vi "Dashboard Main.vi"() -> ()   [LabVIEW 2015]
uses:
  C/Program Files (x86)/National Instruments/LabVIEW 2015/examples/FRC/roboRIO/Vision/2016 Vision Example/Vision Support Code/Camera Types.ctl
  <vilib>/Rock Robotics/WPI/Camera/WPI_CameraSettings Read MJPG.ctl
  <vilib>/Rock Robotics/WPI/Camera/WPI_CameraImageSize.ctl
  <vilib>/Utility/miscctls.llb/LVRowAndColumnTypeDef.ctl
  <vilib>/event_ctls.llb/eventvkey.ctl
  <vilib>/Rock Robotics/WPI/Dashboard/WPI_DashboardLogging Global.vi
  <vilib>/Rock Robotics/Network Tables/NT Write Boolean.vi
  <vilib>/Rock Robotics/Network Tables/NT Read Numeric Array.vi
  <vilib>/Utility/config.llb/Write Key (String).vi
  <vilib>/Utility/config.llb/Write Key (I32).vi
  <vilib>/Utility/config.llb/NI_LVConfig.lvlib
  <vilib>/vision/NI_Vision_Development_Module.lvlib
panel:
  in  "Vision":u16(ring)=1 items=["Camera Off", "USB Camera SW", "USB Camera HW", "IP Camera"]
  out "Camera IP 2":string
  in  "Rec Mode 2":enum32{"Stop", "Record", "Playback"}(radio)
  out "Original Image":T1(plugin-control)
  out "Sorted Particle Scores":T2(array[cluster]) {"Moment Factor" format="%#_3g"; "Aspect Ratio" format="%#_3g"; "Area to CH" format="%#_3g"; "X" format="%#_3g"; "Y" format="%#_3g"}
  out "Detected Targets":T3(array[cluster]) {"Normalized Rect"."Numeric 5" format="%#_2g"; "Normalized Rect"."Numeric 3" format="%#_2g"; "Normalized Rect"."Numeric 2" format="%#_2g"; "Normalized Rect"."Numeric" format="%#_2g"}
  in  "TCP":refnum<k5>
  in  "Rec Mode":enum32{"Stop", "Record", "Playback"}(radio)
  in  "Vision - Dissabled Control":u16(ring)=1 items=["Camera Off", "USB Camera SW", "USB Camera HW", "IP Camera"]
  out "Camera IP":string
  out "Image Message":string="Timeout in Camera Communications"
  in  "Dashboard Tab":T4(tab)
  in  "ACTIVE CAMERA":bool=TRUE
  out "Target Horizontal Degrees":dbl(knob) scale=-30.0..30.0
  out "Target Vertical Angle":dbl(knob) scale=-30.0..30.0
  out "Target Visible":bool
  in  "Camera Address 2":string="USB 0"
  in  "Camera Settings":T5={"fps"=30, "compression"=30, "Image Size"=enum."640x480"}
  out "Auton Mode":string
  in  "Select Auto":string(combo)
  out "NT Connection":bool
  in  "Camera Settings":T7={"Frame Rate"=30, "Compression"=30, "Size"=1} {"Frame Rate" scale=1.0..30.0; "Size" items=["640x480", "320x240", "160x120"]}
  out "MotorChart R":cluster{"Numeric":dbl, "Numeric":dbl}(graph)
  out "MotorChart L":T8(graph)
  out "MotorSliders R":cluster{"MotorSlide1":dbl, "MotorSlide2":dbl} {"MotorSlide2" scale=-1.0..1.0 scale format="%#_2e"; "MotorSlide1" scale=-1.0..1.0 scale format="%#_2e"}
  out "MotorSliders L":T9 {"MotorSlide4 2" scale=0.0..14.0 scale format="%#_2e"; "MotorSlide2" scale=-1.0..1.0 scale format="%#_2e"; "MotorSlide1" scale=-1.0..1.0 scale format="%#_2e"}
  out "Gyro":dbl(knob) scale=0.0..360.0
  out "JS1 Z":dbl(slide) scale=-1.0..1.0 scale format="%#_2e"
  out "JS1 Graph":cluster{"X":dbl, "Y":dbl}[](graph)
  out "JS1 Buttons":T10
  out "JS2 Z":dbl(slide) scale=-1.0..1.0 scale format="%#_2e"
  out "JS2 Graph":cluster{"X":dbl, "Y":dbl}[](graph)
  out "JS2 Buttons":T10
  out "Mode":T11(ring)=enum."Auto Disabled"
  in  "DB Camera Config":bool
  out "fps":dbl format="%#.1g"
  out "Mbps":dbl format="%#.1g"
  out "Mbps LED":bool
  in  "DB/String 9":string
  in  "DB/String 8":string
  in  "DB/String 7":string
  in  "DB/String 6":string
  in  "DB/String 5":string
  in  "DB/String 4":string
  in  "DB/String 3":string
  in  "DB/String 2":string
  in  "DB/String 1":string
  in  "DB/String 0":string
  in  "DB/Slider 0":dbl(slide) scale=0.0..5.0
  in  "DB/Slider 1":dbl(slide) scale=0.0..5.0
  in  "DB/Slider 2":dbl(slide) scale=0.0..5.0
  in  "DB/Slider 3":dbl(slide) scale=0.0..5.0
  out "DB/LED 3":bool
  out "DB/LED 2":bool
  out "DB/LED 1":bool
  out "DB/LED 0":bool
  in  "DB/Button 3":bool
  in  "DB/Button 2":bool
  in  "DB/Button 1":bool
  in  "DB/Button 0":bool caption="New Name"
  in  "LED Color":T12={"Hue"={45.0, 125.0}, "Sat"={0.0, 255.0}, "Val"={250.0, 255.0}} {"Hue" scale=0.0..255.0 scale format="%#_3g"}
  in  "Std Devs for Cal":cluster{"H":dbl, "S":dbl, "V":dbl}={"H"=4.0, "S"=6.0, "V"=4.0}
  in  "Min Score Thresh":i32=60
  out "Highest Avg Score":dbl format="%#_3g"
  in  "Anno Limit":dbl=75.0
  out "Qualified Particles":i32
  out "Masked":T1(plugin-control)
  in  "Green BCG Values (Brightness 1)":T13={"Brightness"=100.0, "Contrast"=45.0, "Gamma"=1.0}
  in  "Annotate":bool=TRUE
  in  "Asp Rat FFact":dbl=1.0
  in  "Emphasize Limit Tests":bool=TRUE
  in  "Camera Type":T14=enum."MS HD3000 640x480"
  in  "Test Slider":dbl(slide) scale=0.0..100.0 scale format="%#_3g"
  in  "On/Off":bool caption="Solenoid"
  in  "Test Name":u16(ring) items=["Select the test to run..."]
  in  "Test Tree":string(tree)
  in  "Motor":cluster{"Value":dbl, "Enable":bool} {"Value" scale=-1.0..1.0 scale format="%#_3g"}
  out "Progress":T15 {"Test Progress" scale=0.0..100.0}
  in  "Rev/Fwd":cluster{"Forward":bool, "Reverse":bool}
  in  "Test Ring":u16(ring) items=["Monochrome", "Color"]
  out "Cmd Status":string
  in  "Execute Command":bool
  in  "Command Params":string[][](table)
  in  "Command Selection":i32(listbox)
  in  "CheckList":i32(listbox)
  out "Tree":string(tree)
  out "Camera Image":T1(plugin-control)
  out "Background":bool
  # "Density Profile"
  # "Left"
  # "Front"
  # "Right"
  # "Battery"
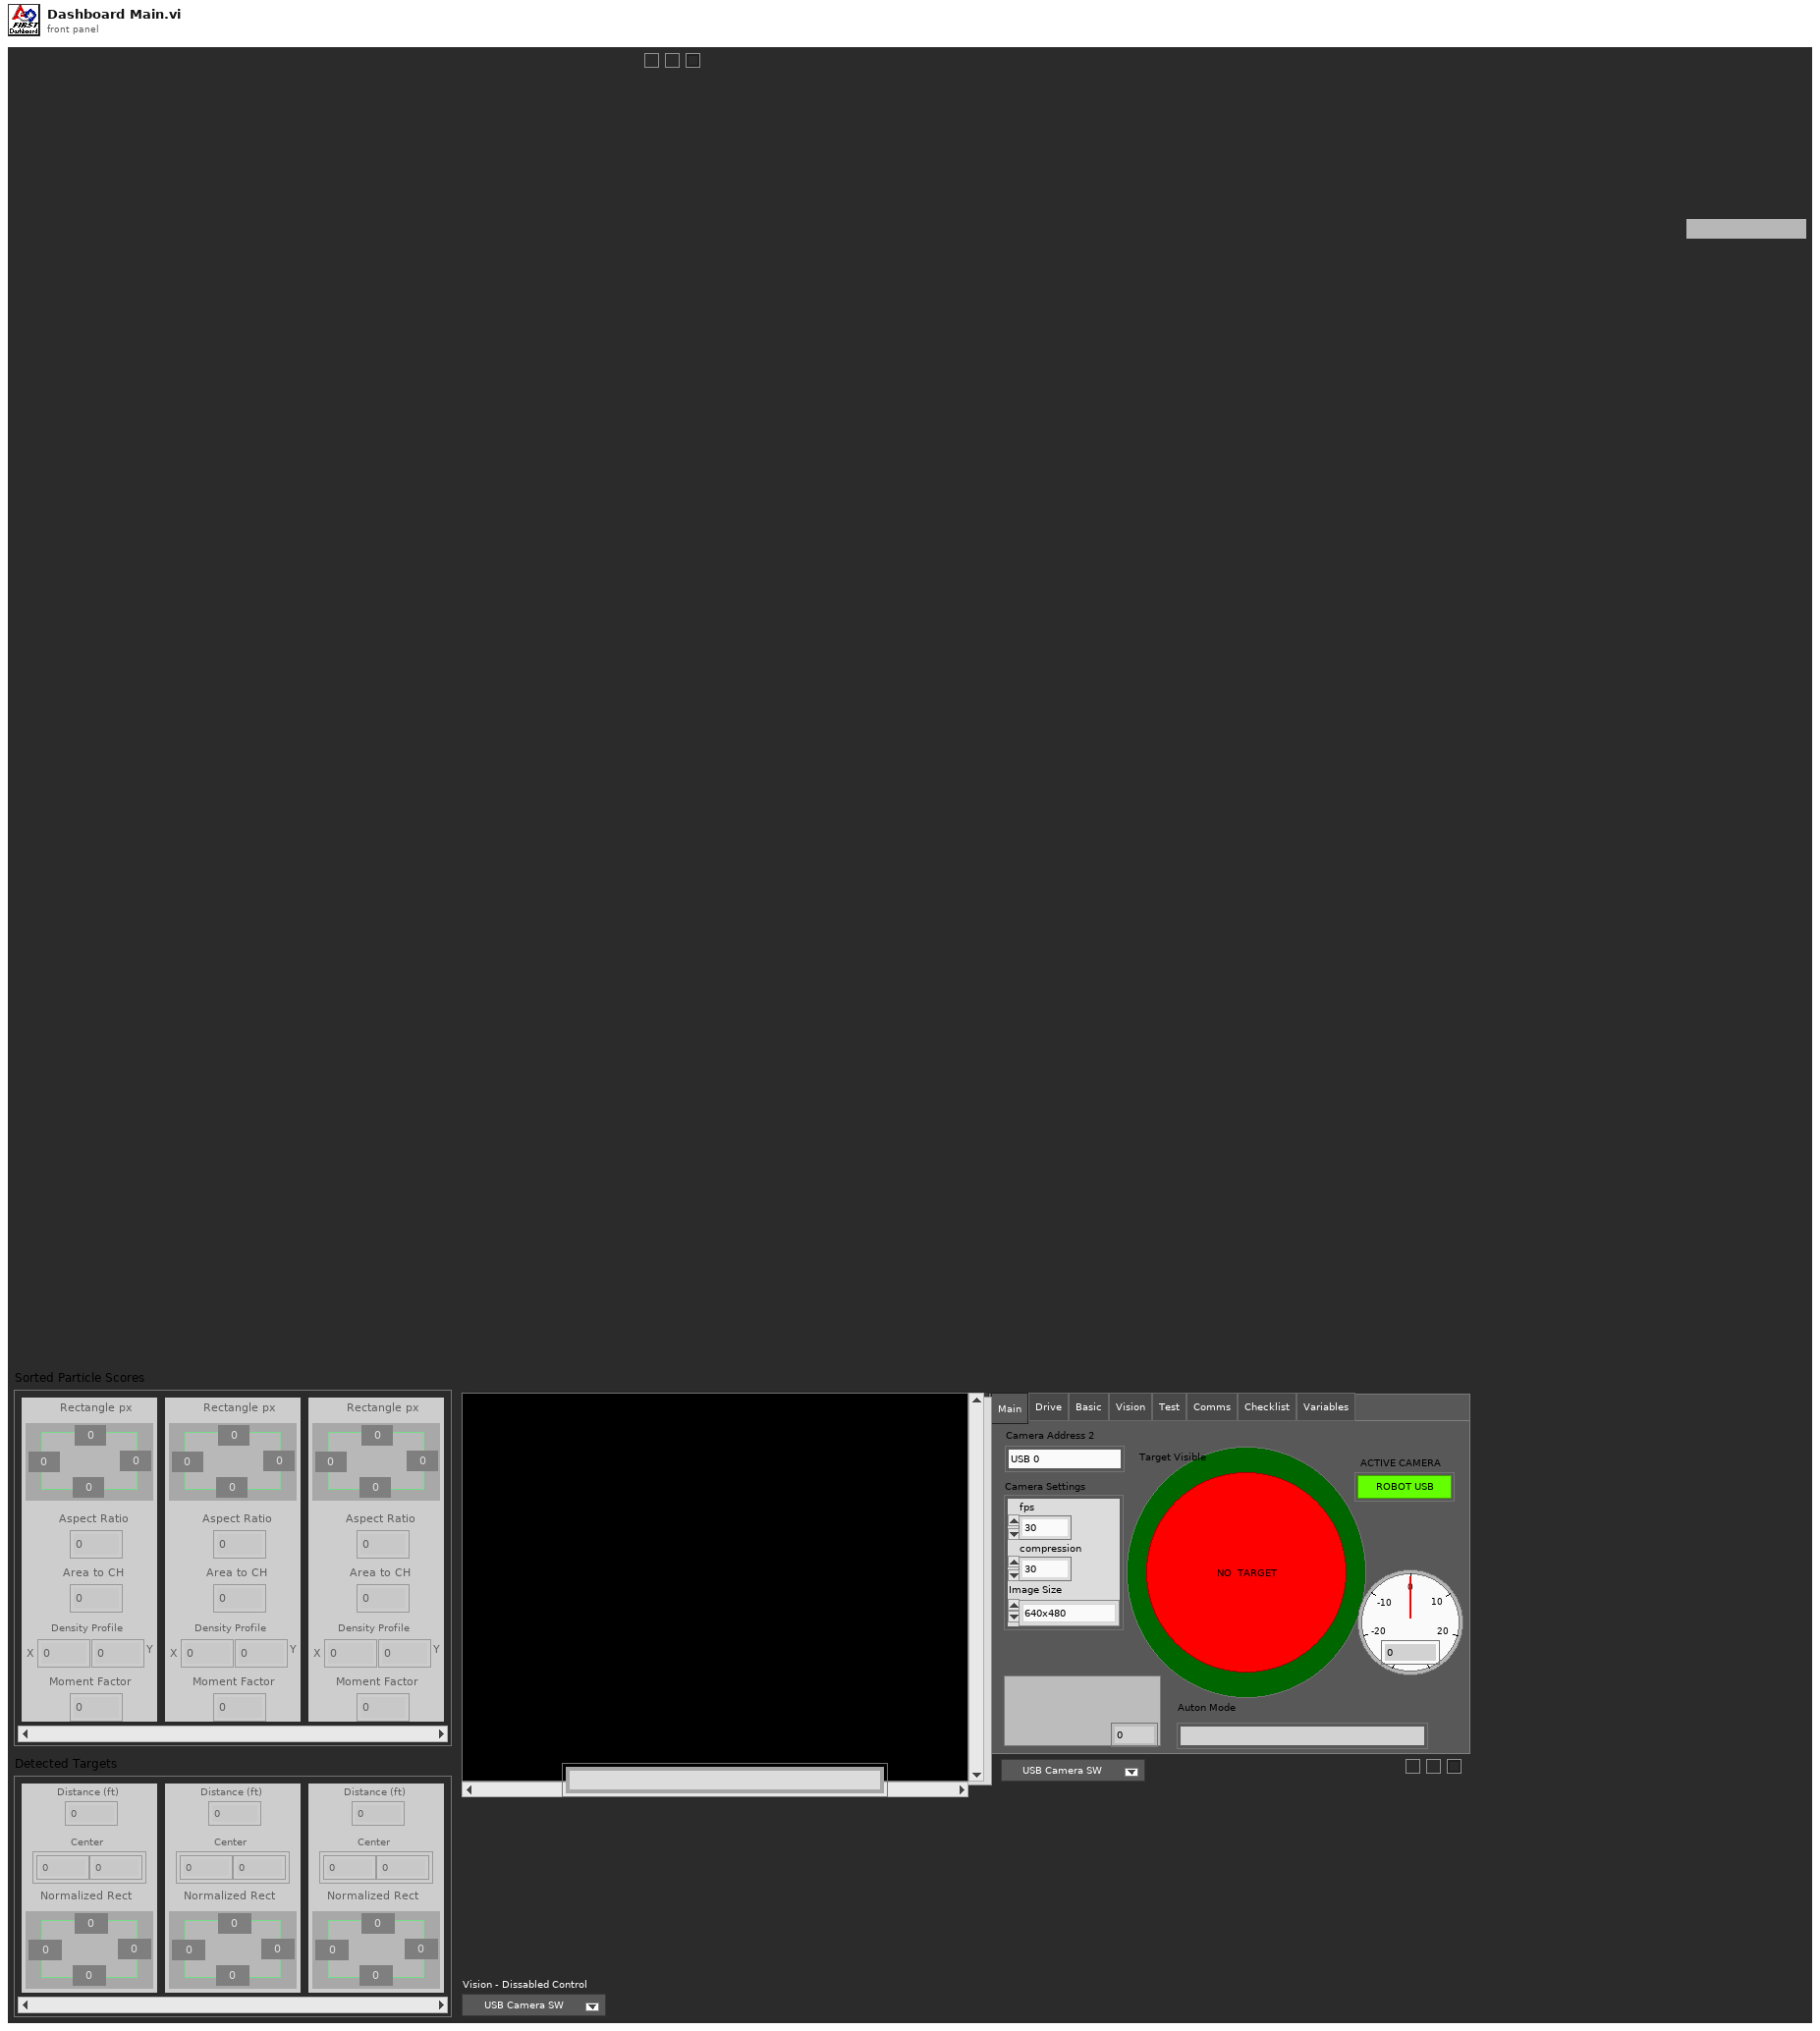
[diagram p1: front panel]
types:
  T1 = typedef "IMAQ Image.ctl" = refnum<image>
  T2 = cluster{"Rectangle px":cluster{"Numeric":dbl, "Numeric 2":dbl, "Numeric 3":dbl, "Numeric 5":dbl}, "Aspect Ratio":dbl, "Area to CH":dbl, "X":dbl, "Y":dbl, "Moment Factor":dbl}[]
  T3 = cluster{"Distance (ft)":dbl, "Center":cluster{dbl, dbl}, "Normalized Rect":cluster{"Numeric":dbl, "Numeric 2":dbl, "Numeric 3":dbl, "Numeric 5":dbl}}[]
  T4 = enum32{"Main", "Drive", "Basic", "Vision", "Test", "Comms", "Checklist", "Variables"}
  T5 = typedef "WPI_CameraSettings Read MJPG.ctl" = cluster{"fps":i32, "compression":i32, "Image Size":T6}
  T6 = typedef "WPI_CameraImageSize.ctl" = enum16{"640x480", "320x240", "160x120", "Custom"}
  T7 = cluster{"Frame Rate":i32, "Compression":i32, "Size":u16}
  T8 = cluster{"Numeric":dbl, "Numeric":dbl, "Battery V":dbl}
  T9 = cluster{"MotorSlide1":dbl, "MotorSlide2":dbl, "MotorSlide4 2":dbl}
  T10 = cluster{bool, bool, bool, bool, bool, bool, bool, bool, bool, bool, bool, bool}
  T11 = enum8{"Tele-Op Disabled", "Tele-Op Enabled", "Auto Disabled", "Auto Enabled", "Test Disabled", "Test Enabled", "Disconnected", "No Code", "E-Stop"}
  T12 = cluster{"Hue":cluster{dbl, dbl}, "Sat":cluster{dbl, dbl}, "Val":cluster{dbl, dbl}}
  T13 = cluster{"Brightness":sgl, "Contrast":sgl, "Gamma":sgl}
  T14 = typedef "Camera Types.ctl" = enum16{"206", "1011", "1013", "MS HD3000 square", "MS HD3000 640x480"}
  T15 = cluster{"Test Progress":u8, "Test Progress Text":string}
  T16 = typedef "Particle Parameters" = i32
  T17 = typedef "Image Type" = u32
  T18 = cluster{"IDs":cluster{"RPC field ID":u16, "Unique ID":u16}, "String":string}
  T19 = enum32{"Drive", "Basic", "Custom", "Test", "Checklist", "Variables"}
  T20 = cluster{"Camera Image":refnum<vi>, "Dashboard Tab":refnum<vi>, "Background":refnum<vi>, "Vision - Dissabled Control":refnum<vi>, "Rec Mode":refnum<vi>, "Test Slider":refnum<vi>, "On/Off ":refnum<vi>, "Test Ring":refnum<vi>, "Rev/Fwd":refnum<vi>, "Test Name":refnum<vi>, "Motor":refnum<vi>, "Progress":refnum<vi>, "CheckList":refnum<vi>, "Tree":refnum<vi>, "Test Tree":refnum<vi>, "Command Params":refnum<vi>, "Command Selection":refnum<vi>, "Execute Command":refnum<vi>, "Cmd Status":refnum<vi>}
  T21 = cluster{cluster{dbl, dbl}, cluster{dbl, dbl}, cluster{dbl, dbl}}
  T22 = cluster{"Bounding box":cluster{"left":dbl, "top":dbl, "right":dbl, "bottom":dbl}, "Aspect Ratio":dbl, "Area to CH":dbl, "X Mask":dbl, "Y Mask":dbl, "Moment":dbl}[]
  T23 = cluster{"Rectangle":cluster{"Numeric":dbl, "Numeric 2":dbl, "Numeric 3":dbl, "Numeric 5":dbl}, "L":dbl, "Area to CH":dbl, "X":dbl, "Y":dbl, "Moment Factor":dbl}[]
  T24 = cluster{"Distance (ft)":dbl, "Center":cluster{dbl, dbl}, "Normalized Rect":cluster{"Numeric":dbl, "Numeric 2":dbl, "Numeric 3":dbl, "Numeric 5":dbl}}
  T25 = cluster{"Rectangle":cluster{"Numeric":dbl, "Numeric 2":dbl, "Numeric 3":dbl, "Numeric 5":dbl}, "L":dbl, "Area to CH":dbl, "X":dbl, "Y":dbl, "Moment Factor":dbl}
  T26 = cluster{"Numeric":dbl, "Numeric 2":dbl, "Numeric 3":dbl, "Numeric 5":dbl}
  T27 = cluster{"Error Strings":string, "Disable Counts":cluster{u16, u16}, "Rail Faults":cluster{u16, u16, u16}, "Robot IP":string, "DB Mode":u8, "Event Info":cluster{"Name":string, "Type":u8, "Number":u16, "Replay":u8}, "Camera Addr":string}
  T28 = cluster{"Storage":cluster{"Disk Free":u64, "RAM Block":u32, "RAM free":u32}, "CPU Utilization":cluster{"CPU % ISR":sgl, "CPU % Time Crit":sgl, "CPU % Timed Str":sgl, "CPU % High":sgl, "CPU % Above":sgl, "CPU % Normal":sgl, "CPU % Low":sgl}, "CAN":cluster{"% Bus Utilization":sgl, "Bus Off Cnt":u32, "TX_FIFO Full Cnt":u32, "Receive Error Cnt":u8, "Transmit Error Cnt":u8}, "HID":cluster{"HID Outputs":u32, "Rumble Low":u16, "Rumble High":u16}[]}
  T29 = cluster{"Status bits":cluster{"Test Mode":bool, "Autonomous":bool, "Enabled":bool, "Code Start":bool, "Brownout":bool, "Reserved 2":bool, "Reserved 3":bool, "E-Stop":bool}, "Code Trace":cluster{"Disabled":bool, "TeleOp":bool, "Auto":bool, "Test":bool}, "Controller Type":enum16{"unknown", "cRIO", "roboRio"}, "Code?":enum16{"unknown", "noCode", "code"}, "Battery V":dbl}
  T30 = cluster{"Control Bits":cluster{"TestMode":bool, "Autonomous":bool, "Enabled":bool, "FMS Present":bool, bool, bool, bool, "E-Stop":bool}, "Team Station ":u8, "Countdown":sgl, "Joystick Values":cluster{"Axes":dbl[], "Buttons":bool[], "POVs":i16[]}[]}
  T31 = cluster{"Axes":dbl[], "Buttons":bool[], "POVs":i16[]}[]
  T32 = cluster{"Axes":dbl[], "Buttons":bool[], "POVs":i16[]}
  T33 = cluster{"Buttons[0]":bool, "Buttons[1]":bool, "Buttons[2]":bool, "Buttons[3]":bool, "Buttons[4]":bool, "Buttons[5]":bool, "Buttons[6]":bool, "Buttons[7]":bool, "Buttons[8]":bool, "Buttons[9]":bool, "Buttons[10]":bool, "Buttons[11]":bool}
  T34 = typedef "NI_LVConfig.lvlib/Config Data RefNum.ctl" = refnum<k1>
  T35 = cluster{"Operation":enum16{"Update", "Clear"}, "Color Box":u32}[]
  T36 = typedef "eventvkey.ctl" = enum16{"ASCII", "Enter", "Return", "Shift", "Ctrl", "Alt", "Cmd", "Opt", "Caps", "NumLock", "Clear", "Break", "Up", "Down", "Left", "Right", "Insert", "Delete", "Home", "End", "PageUp", "PageDown", "Escape", "Help", "Pause", "ScrollLock", "F1", "F2", "F3", "F4", "F5", "F6", "F7", "F8", "F9", "F10", "F11", "F12", "F13", "F14", "F15", "F16", "F17", "F18", "F19", "F20", "F21", "F22", "F23", "F24", "Play", "VolumeUp", "VolumeDown", "Mute", "Two Byte Char"}
  T37 = cluster{"Image Size":bool, "Image Type":bool, "Pixel Value":bool, "ROI Information":bool, "Zoom Factor":bool}
  T38 = enum8{"Enabled", "Disabled", "Disabled and Grayed Out"}
  T39 = cluster{"Operation":enum16{"Update", "Clear"}, "Color Box":u32}
  T40 = typedef "LVRowAndColumnTypeDef.ctl" = cluster{"Row":i32, "Column":i32}
  T41 = cluster{"Shift":bool, "Ctrl":bool, "Alt":bool, "Cmd":bool, "Opt":bool}
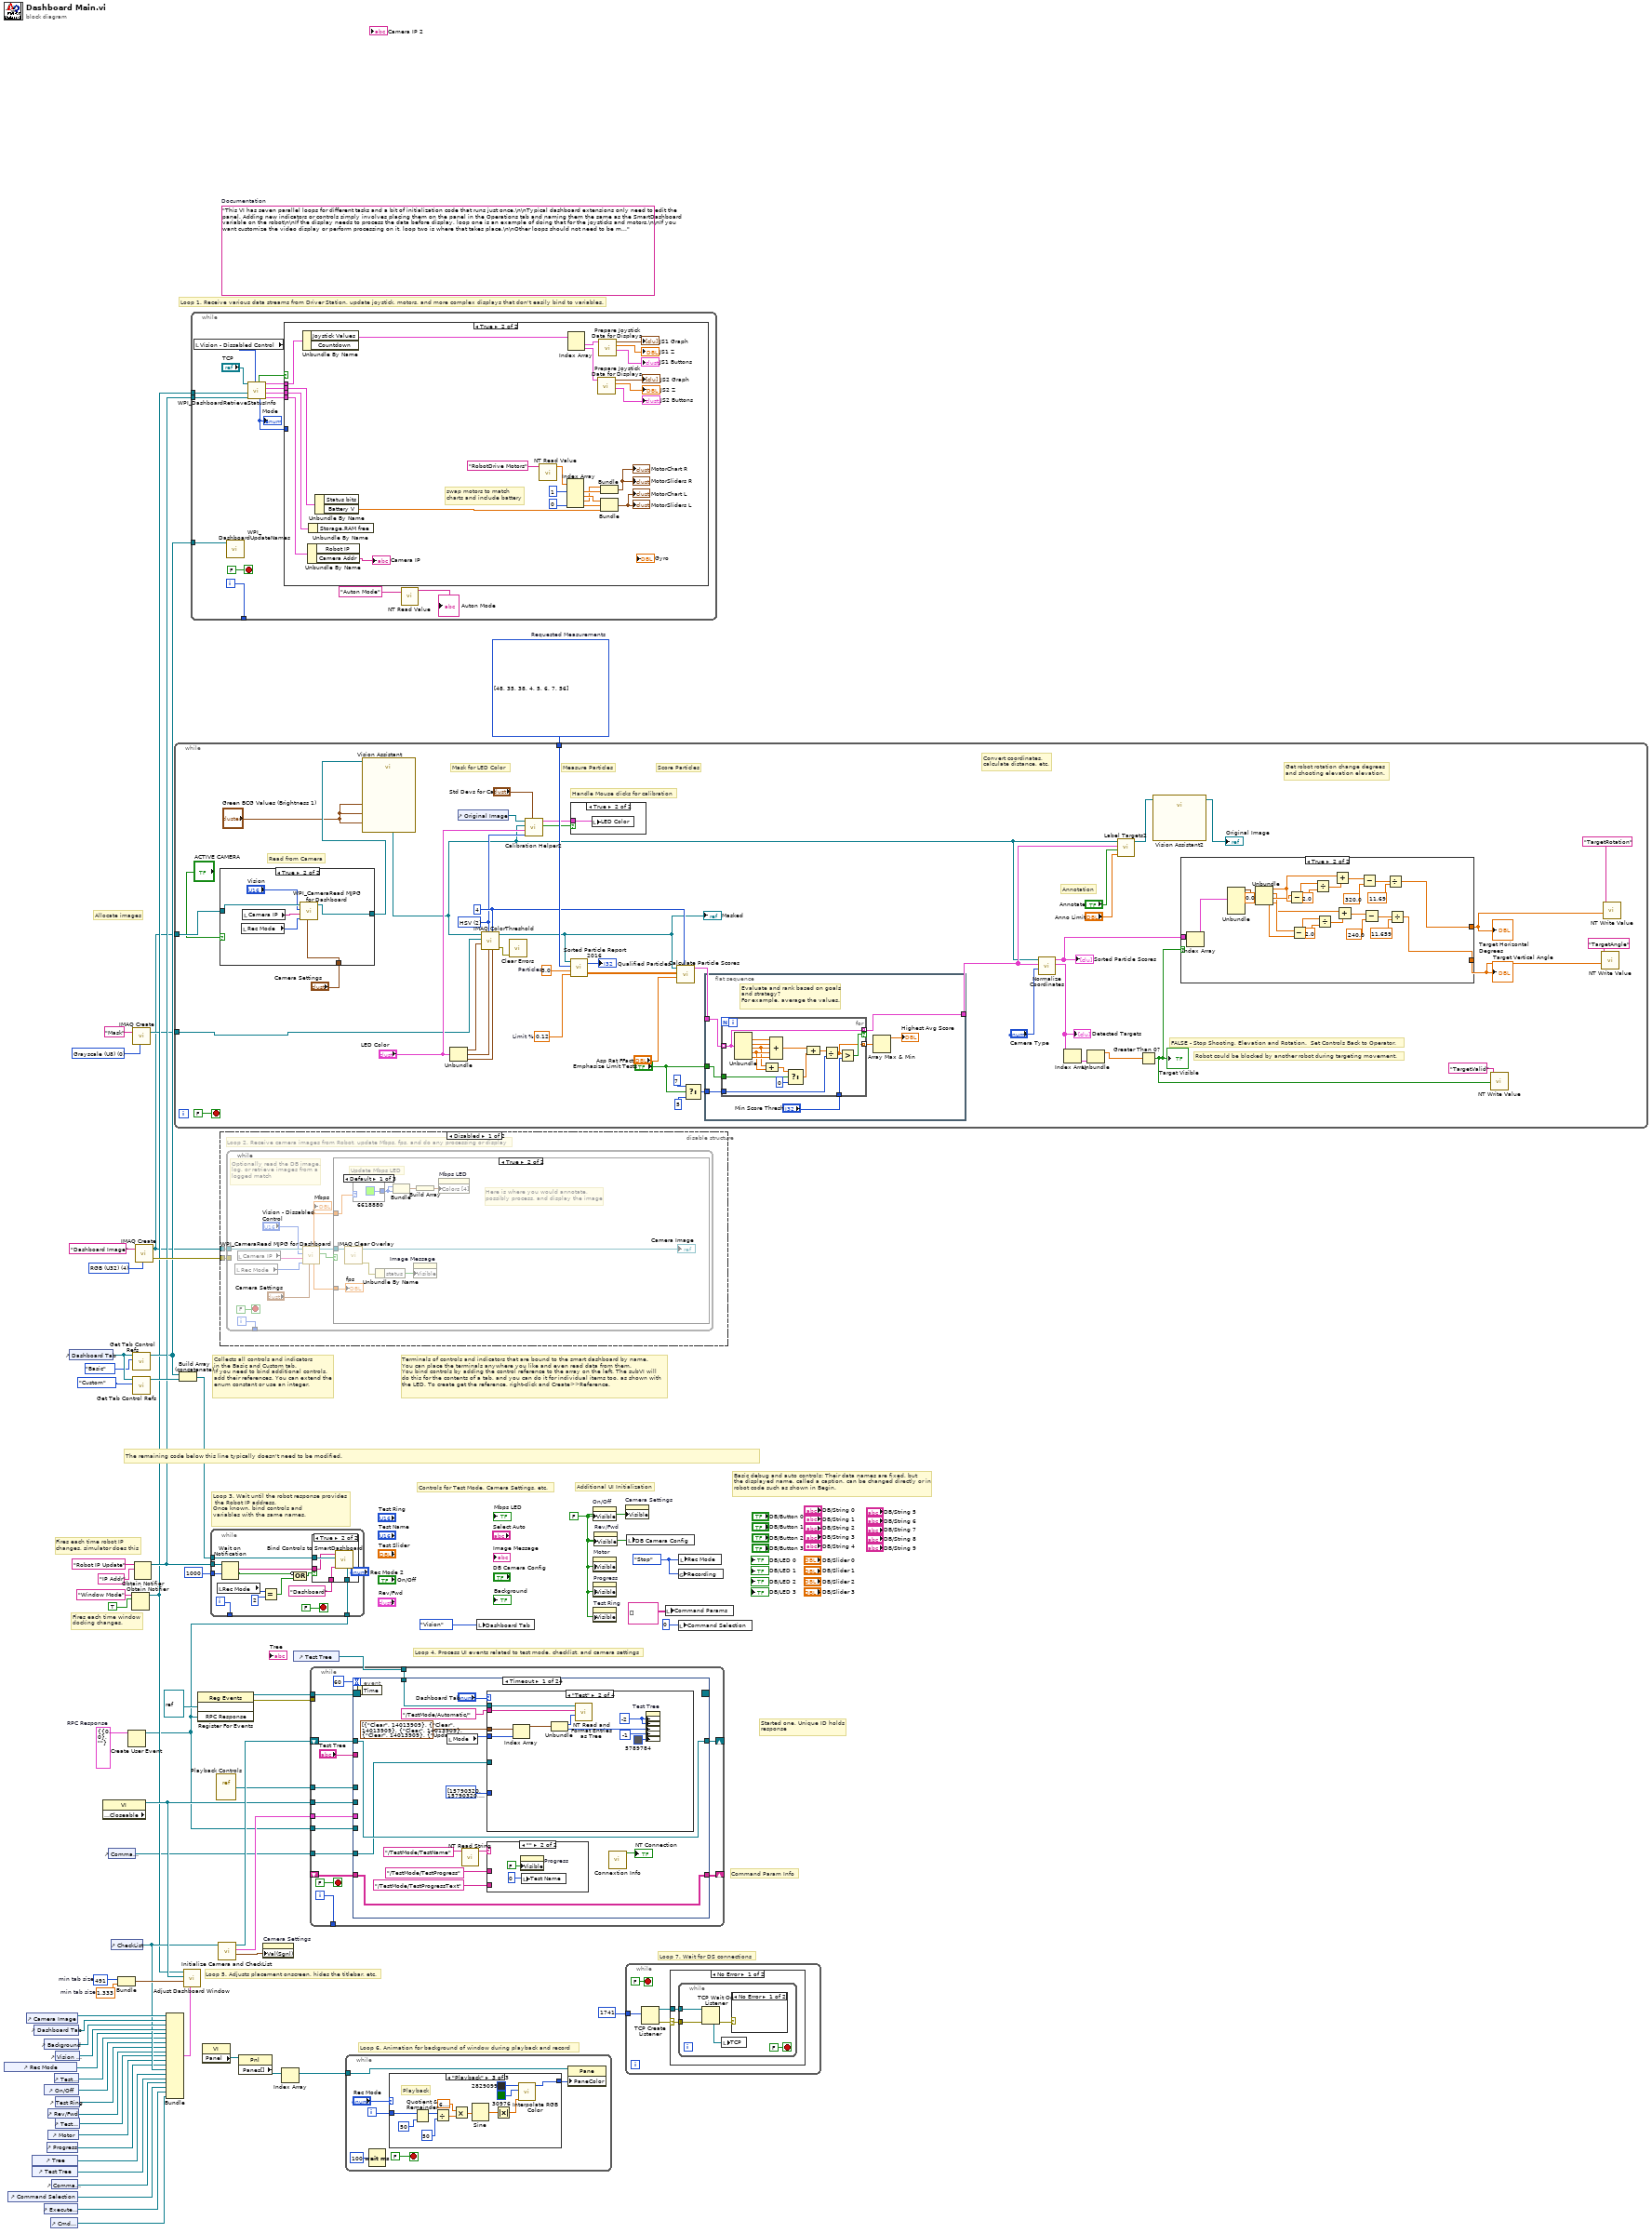
[diagram p0: block diagram]
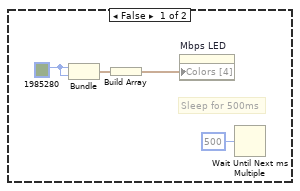
[diagram p2: hidden frame]
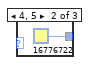
[diagram p3: hidden frame]
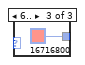
[diagram p4: hidden frame]
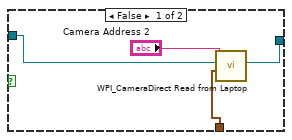
[diagram p6: hidden frame]
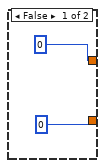
[diagram p7: hidden frame]
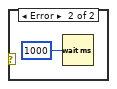
[diagram p9: hidden frame]
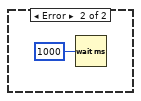
[diagram p10: hidden frame]
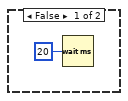
[diagram p11: hidden frame]
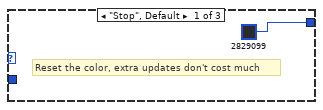
[diagram p12: hidden frame]
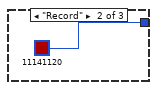
[diagram p13: hidden frame]
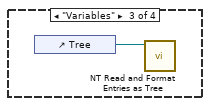
[diagram p16: hidden frame]
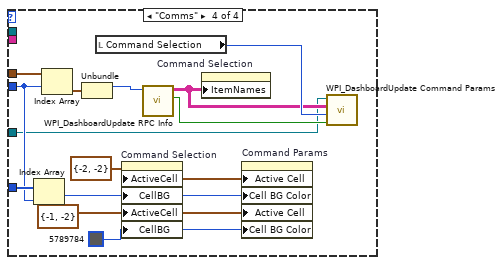
[diagram p17: hidden frame]
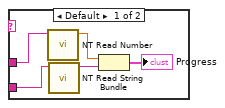
[diagram p18: hidden frame]
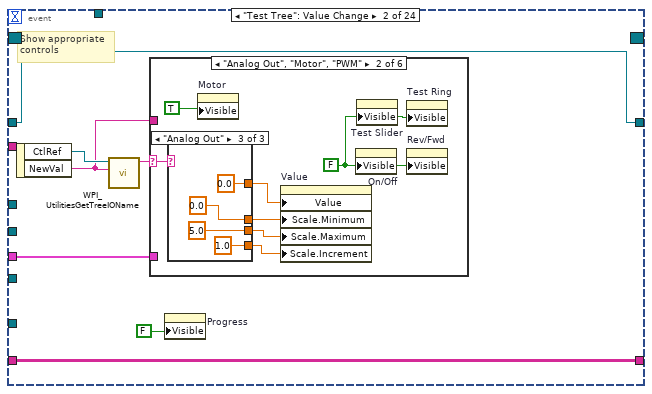
[diagram p19: hidden frame]
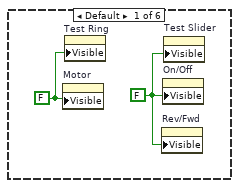
[diagram p20: hidden frame]
diagram:
  w2 = T16[] [48, 35, 38, 4, 5, 6, 7, 56] items=["Center of Mass X", "Center of Mass Y", "First Pixel X", "First Pixel Y", "Bounding Rect Left", "Bounding Rect Top", "Bounding Rect Right", "Bounding Rect Bottom", "Max Feret Diameter Start X", "Max Feret Diameter Start Y", "Max Feret Diameter End X", "Max Feret Diameter End Y", "Max Horiz. Segment Length Left", "Max Horiz. Segment Length Right", "Max Horiz. Segment Length Row", "-", "Bounding Rect Width", "Bounding Rect Height", "Bounding Rect Diagonal", "Perimeter", "Convex Hull Perimeter", "Holes' Perimeter", "Max Feret Diameter", "Equivalent Ellipse Major Axis", "Equivalent Ellipse Minor Axis", "Equivalent Ellipse Minor Axis (Feret)", "Equivalent Rect Long Side", "Equivalent Rect Short Side", "Equivalent Rect Diagonal", "Equivalent Rect Short Side (Feret)", "Average Horiz. Segment Length", "Average Vert. Segment Length", "Hydraulic Radius", "Waddel Disk Diameter", "-", "Area", "Holes' Area", "Particle & Holes' Area", "Convex Hull Area", "Image Area", "-", "Number of Holes", "Number of Horiz. Segments", "Number of Vert. Segments", "-", "Orientation", "Max Feret Diameter Orientation", "-", "% Area/Image Area", "% Area/(Particle & Holes' Area)", "Ratio of Equivalent Ellipse Axes", "Ratio of Equivalent Rect Sides", "-", "Elongation Factor", "Compactness Factor", "Heywood Circularity Factor", "Type Factor", "-", "Sum X", "Sum Y", "Sum XX", "Sum XY", "Sum YY", "Sum XXX", "Sum XXY", "Sum XYY", "Sum YYY", "-", "Moment of Inertia XX", "Moment of Inertia XY", "Moment of Inertia YY", "Moment of Inertia XXX", "Moment of Inertia XXY", "Moment of Inertia XYY", "Moment of Inertia YYY", "Norm. Moment of Inertia XX", "Norm. Moment of Inertia XY", "Norm. Moment of Inertia YY", "Norm. Moment of Inertia XXX", "Norm. Moment of Inertia XXY", "Norm. Moment of Inertia XYY", "Norm. Moment of Inertia YYY", "Hu Moment 1", "Hu Moment 2", "Hu Moment 3", "Hu Moment 4", "Hu Moment 5", "Hu Moment 6", "Hu Moment 7"]  # Requested Measurements
  w5 = T17 0 items=["Grayscale (U8)", "Grayscale (I16)", "Grayscale (SGL)", "Complex (CSG)", "RGB (U32)", "HSL (U32)", "RGB (U64)", "Grayscale (U16)"] ("Image Type")
  w12 = T18 {"IDs"={"RPC field ID"=0, "Unique ID"=0}, "String"=""}  # RPC Response
  w38 = 491  # min tab size
  w37 = 1.333  # min tab size
  w46 = enum32{"Stop", "Record", "Playback"}."Stop" ("Rec Mode")
  w20 = FALSE ("Visible")
  (unwired) "This VI has seven parallel loops for different tasks and a bit of initialization code that runs just once.\n\nTypical dashboard extensions only need to edit the panel. Adding new indicators or controls simply involves placing them on the panel in the Operations tab and naming them the same as the SmartDashboard variable on the robot\n\nIf the display needs to process the data before display, loop one is an example of doing that for the joysticks and motors.\n\nIf you want customize the video display or perform processing on it, loop two is where that takes place.\n\nOther loops should not need to be modified. They are pretty standard, and document the task they perform."  # Documentation
  w65 = T17 4 items=["Grayscale (U8)", "Grayscale (I16)", "Grayscale (SGL)", "Complex (CSG)", "RGB (U32)", "HSL (U32)", "RGB (U64)"] ("Image Type")
  # "Allocate images"
  # "Command Param Info"
  # "Started one, Unique ID holds\nresponse"
  # "Loop 7. Wait for DS connections"
  # "Basic debug and auto controls: Their data names are fixed, but\nthe displayed name, called a caption, can be changed directly or in\nrobot code such as shown in Begin."
  # "Controls for Test Mode, Camera Settings, etc."
  # "Additional UI Initialization"
  # "Loop 6. Animation for background of window during playback and record"
  # "Fires each time robot IP\nchanges, simulator does this"
  # "Fires each time window\ndocking changes."
  # "Collects all controls and indicators\nin the Basic and Custom tab.\nIf you need to bind additional controls,\nadd their references. You can extend the\nenum constant or use an integer."
  # "The remaining code below this line typically doesn't need to be modified."
  # "Loop 4. Process UI events related to test mode, checklist, and camera settings"
  # "Terminals of controls and indicators that are bound to the smart dashboard by name.\nYou can place the terminals anywhere you like and even read data from them.\nYou bind controls by adding the control reference to the array on the left. The subVI will\ndo this for the contents of a tab, and you can do it for individual items too, as shown with\nthe LED. To create get the reference, right-click and Create>>Reference."
  # "Loop 3. Wait until the robot response provides\n the Robot IP address.\nOnce known, bind controls and\nvariables with the same names."
  # "Loop 5. Adjusts placement onscreen, hides the titlebar, etc."
  # "Loop 1. Receive various data streams from Driver Station, update joystick, motors, and more complex displays that don't easily bind to variables."
  n1 = control-ref of="Rec Mode"() -> (w26:refnum<vi>)
  n2 = control-ref of="Command Selection"() -> (w11:refnum<vi>)
  n3 = control-ref of="Camera Image"() -> (w41:refnum<vi>)
  n4 = control-ref of="Tree"() -> (w30:refnum<vi>)
  n5 = control-ref of="Test Tree"() -> (w29:refnum<vi>)
  n6 = control-ref of="Dashboard Tab"() -> (w40:refnum<vi>)
  n7 = control-ref of="Execute Command"() -> (w13:refnum<vi>)
  n8 = control-ref of="Background"() -> (w35:refnum<vi>)
  n9 = control-ref of="On/Off"() -> (w24:refnum<vi>)
  n10 = control-ref of="Progress"() -> (w21:refnum<vi>)
  n11 = control-ref of="Rev/Fwd"() -> (w22:refnum<vi>)
  n12 = control-ref of="Motor"() -> (w27:refnum<vi>)
  n13 = control-ref of="Cmd Status"() -> (w7:refnum<vi>)
  n14 = control-ref of="Command Params"() -> (w14:refnum<vi>)
  n15 = control-ref of="Test Slider"() -> (w25:refnum<vi>)
  n16 = control-ref of="Vision - Dissabled Control"() -> (w39:refnum<vi>)
  n17 = control-ref of="Test Ring"() -> (w23:refnum<vi>)
  n18 = control-ref of="Test Name"() -> (w28:refnum<vi>)
  n19 = control-ref of="Dashboard Tab"() -> (w44:refnum<vi>)
  n20 = property class="VI" props=["Front Panel.Closeable"]() -> (reference out=w45:refnum<vi>)  [unwired: 2 in, 2 out]
  n21 = control-ref of="Command Params"() -> (w6:refnum<vi>)
  n22 = control-ref of="CheckList"() -> (w31:refnum<vi>)
  n23 = Bundle("min tab size"=w38, "min tab size"=w37) -> (w36:cluster{"min tab size":i32, "min tab size":dbl})  [unwired: 1 in]
  n24 = Create User Event(user event datatype=w12) -> (user event=w8:refnum<user-event>)  [unwired: 1 in, 1 out]
  n25 = Obtain Notifier(name (unnamed)="Window Mode", notification data type=TRUE) -> (notifier out=w17:refnum<notifier>)  [unwired: 2 in, 2 out]
  n26 = call "IMAQ Create"("Image Name"="Mask", "Image Type"=w5) -> ("New Image"=w3:T1)  [unwired: 2 in, 2 out]
  n27 = call <vilib>:"Get Tab Control Refs.vi"("Page Index"=T19."Basic" ("Dashboard Tab"), "TabControl in"=w44) -> ("ControlsOnPage"=w18:refnum<vi>[])  [unwired: 9 in]
  n28 = call <vilib>:"Get Tab Control Refs.vi"("Page Index"=T19."Custom" ("Dashboard Tab"), "TabControl in"=w44) -> ("ControlsOnPage"=w43:refnum<vi>[])  [unwired: 9 in]
  n29 = Obtain Notifier(name (unnamed)="Robot IP Update", notification data type="IP Addr" ("name (unnamed)")) -> (notifier out=w19:refnum<notifier>)  [unwired: 2 in, 2 out]
  n30 = call "IMAQ Create"("Image Name"="Dashboard Image", "Image Type"=w65) -> ("New Image"=w1:T1, "error out"=w63:errorcluster)  [unwired: 2 in, 1 out]
  n31 = Bundle("Camera Image"=w41, "Dashboard Tab"=w40, "Background"=w35, "Vision - Dissabled Control"=w39, "Rec Mode"=w26, "Test Slider"=w25, "On/Off"=w24, "Test Ring"=w23, "Rev/Fwd"=w22, "Test Name"=w28, "Motor"=w27, "Progress"=w21, "CheckList"=w31, "Tree"=w30, "Test Tree"=w29, "Command Params"=w14, "Command Selection"=w11, "Execute Command"=w13, "Cmd Status"=w7) -> (w32:T20)  [unwired: 1 in]
  n32 = while {
    tunnel: w1 -> [w72]
    tunnel: w3 -> [w74]
    tunnel: w2 -> [w108]
    stop <- FALSE stop-if-true
    w102 = 4 ("Replace Value")
    w104 = 0.12  # Limit %
    w107 = 3.0  # Particles
    w88 = u16 2 items=["RGB", "HSL", "HSV", "HSI"] ("Color Mode")
    # "Read from Camera"
    # "Robot could be blocked by another robot during targeting movement."
    # "Get robot rotation change degrees \nand shooting elevation elevation."
    # "FALSE - Stop Shooting, Elevation and Rotation.  Set Controls Back to Operator."
    # "Handle Mouse clicks for calibration"
    # "Measure Particles"
    # "Convert coordinates,\ncalculate distance, etc."
    # "Annotation"
    # "Score Particles"
    # "Mask for LED Color"
    n33 = case shown="True" "ACTIVE CAMERA" {
      tunnel: w72 -> [w115 w122]
      tunnel: [w114 w121] -> w71
      tunnel: "Camera Settings" -> [w113 w117]
      frame False {
        n34 = call <vilib>:"WPI_CameraDirect Read from Laptop.vi"("Camera Settings"=w113, "Image"=w115, "address"="Camera Address 2") -> ("Image Out"=w114:T1)  [unwired: 7 in, 1 out]
      }
      frame True {
        n35 = local read "Rec Mode"() -> (w119:enum32{"Stop", "Record", "Playback"})
        n36 = local read "Camera IP"() -> (w120:string)
        n37 = call <vilib>:"WPI_CameraRead MJPG for Dashboard.vi"("Camera Settings"=w117, "Rec Mode"=w119, "Camera IP"=w120, "Camera Mode"="Vision", "Refnum in"=w122) -> ("Refnum out"=w121:T1)  [unwired: 3 in, 3 out]
      }
    }
    n38 = call "Vision Assistant"("Image In"=w71, "Red BCG Values (Brightness 1)"="Green BCG Values (Brightness 1)", "Green BCG Values (Brightness 1)"="Green BCG Values (Brightness 1)", "Blue BCG Values (Brightness 1)"="Green BCG Values (Brightness 1)") -> ("Image Out"=w73:T1)  [unwired: 22 in, 1 out]
    n39 = Unbundle("LED Color") -> ("Hue"=w111:cluster{dbl, dbl}, "Sat"=w110:cluster{dbl, dbl}, "Val"=w109:cluster{dbl, dbl})
    n40 = control-ref of="Original Image"() -> (w91:refnum<vi>)
    n41 = call "IMAQ ColorThreshold"("Blue or Luma or Val or Inten Range"=w109, "Replace Value"=w102, "Green or Sat Range"=w110, "Color Mode"=w88, "Red or Hue Range"=w111, "Image Dst"=w74, "Image Src"=w73) -> ("error out"=w95:errorcluster, "Image Dst Out"=w96:T1)  [unwired: 3 in]
    "Masked" <- w96
    n42 = call <vilib>:"Clear Errors.vi"("error in (no error)"=w95) -> ()  [unwired: 5 in, 2 out]
    n43 = call "Calibration Helper2.vi"("Std Devs"="Std Devs for Cal", "Color Mode"=w88, "Color Components"="LED Color", "Image"=w73, "Image Ctl Refnum"=w91) -> ("Changed"=w90:bool, "output color"=w89:T21)  [unwired: 5 in]
    n44 = call "Sorted Particle Report 2016.vi"("Min Area Size %"=w104, "Particle Count Limit"=w107, "Pixel Measurements"=w108, "Image in"=w96) -> ("Sorted Data"=w105:dbl[][], "Particles"=→"Qualified Particles":i32)
    n45 = case shown="True" w90 {
      tunnel: w89 -> [_ w148]
      frame False {
      }
      frame True {
        n46 = local write "LED Color"(w148) -> ()
      }
    }
    n47 = call "Calculate Particle Scores.vi"("Pixel Value"=w102, "Aspect Fudge Factor"="Asp Rat FFact", "Sorted Data"=w105, "Image in"=w96) -> ("Scores"=w99:T22)  [unwired: 7 in]
    n48 = Select(t=7, s="Emphasize Limit Tests", f=5) -> (s? t:f=w92:i32)
    n49 = flat-sequence {
      tunnel: w99 -> [w154]
      tunnel: [w155] -> w97
      tunnel: w92 -> [w151]
      tunnel: "Emphasize Limit Tests" -> [w149]
      frame #0 {
        # "Evaluate and rank based on goals\nand strategy?\nFor example, average the values."
        n50 = for {
          tunnel: w154 -> [w169] mode=indexing
          tunnel: [w169] -> w155 mode=indexing if=w168
          tunnel: [w167] -> w153 mode=indexing
          tunnel: w151 -> [w166]
          tunnel: "Min Score Thresh" -> [w165]
          tunnel: w149 -> [w158]
          n51 = Unbundle(w169) -> ("Aspect Ratio"=w171:dbl, "Area to CH"=w170:dbl, "X Mask"=w160:dbl, "Y Mask"=w161:dbl, "Moment"=w162:dbl)  [unwired: 1 out]
          n52 = Compound Arithmetic op=ADD(w160, w161) -> (w159:dbl)
          n53 = Compound Arithmetic op=ADD(w171, w170, w160, w161, w162) -> (w164:dbl)
          n54 = Select(t=w159, s=w158, f=0) -> (s? t:f=w157:dbl)
          n55 = Compound Arithmetic op=ADD(w164, w157) -> (w163:dbl)
          n56 = Divide(x=w163, y=w166) -> (x/y=w167:dbl)
          n57 = Greater?(x=w167, y=w165) -> (0:w168:bool)
        }
        n58 = Array Max & Min(array=w153) -> (max value=→"Highest Avg Score":dbl)  [unwired: 3 out]
      }
    }
    n59 = call "Normalize Coordinates.vi"("Camera Type"="Camera Type", "Targets"=w97, "Image in"=w73) -> ("Found Targets"=w84:T3, "Sorted Scores"=w82:T23)  [unwired: 7 in]
    "Sorted Particle Scores" <- w82
    "Detected Targets" <- w84
    n60 = Index Array(array=w84) -> (element=w75:T24)  [unwired: 1 in]
    n61 = Unbundle(w75) -> ("Distance (ft)"=w83:dbl)  [unwired: 2 out]
    n62 = call "Label Targets2.vi"("Score Threshold"="Anno Limit", "Annotate"="Annotate", "Targets"=w97, "Image in"=w73) -> ("Image out"=w68:T1)  [unwired: 7 in]
    n63 = Greater Than 0?(x=w83) -> (x > 0?=w80:bool)
    "Target Visible" <- w80
    n64 = call "Vision Assistant2"("Image In"=w68) -> ("Image Out"=→"Original Image":T1)  [unwired: 25 in, 1 out]
    n65 = case shown="True" w80 {
      tunnel: w82 -> [_ w137]
      tunnel: [0 w136] -> w76
      tunnel: [0 w127] -> w77
      frame False {
      }
      frame True {
        (unwired) 0.0 ("Numeric 3")
        n66 = Index Array(array=w137) -> (element=w138:T25)  [unwired: 1 in]
        n67 = Unbundle(w138) -> ("Rectangle"=w139:T26)  [unwired: 5 out]
        n68 = Unbundle(w139) -> ("Numeric"=w147:dbl, "Numeric 2"=w126:dbl, "Numeric 3"=w128:dbl, "Numeric 5"=w125:dbl)
        n69 = Subtract(x=w128, y=w147) -> (x-y=w143:dbl)
        n70 = Subtract(x=w126, y=w125) -> (x-y=w132:dbl)
        n71 = Divide(x=w143, y=2.0) -> (x/y=w146:dbl)
        n72 = Divide(x=w132, y=2.0) -> (x/y=w129:dbl)
        n73 = Add(x=w147, y=w146) -> (x+y=w145:dbl)
        n74 = Add(x=w125, y=w129) -> (x+y=w130:dbl)
        n75 = Subtract(x=w145, y=320.0) -> (x-y=w144:dbl)
        n76 = Subtract(x=w130, y=240.0) -> (x-y=w131:dbl)
        n77 = Divide(x=w144, y=11.69) -> (x/y=w136:dbl)
        n78 = Divide(x=w131, y=11.659) -> (x/y=w127:dbl)
      }
    }
    "Target Vertical Angle" <- w77
    "Target Horizontal Degrees" <- w76
    n79 = call-poly <vilib>:"NT Write Value.vi"("Boolean"=w80, "Name"="TargetValid") -> ()  [unwired: 9 in, 1 out]
    n80 = call-poly <vilib>:"NT Write Value.vi"("Numeric"=w77, "Name"="TargetAngle") -> ()  [unwired: 9 in, 1 out]
    n81 = call-poly <vilib>:"NT Write Value.vi"("Numeric"=w76, "Name"="TargetRotation") -> ()  [unwired: 9 in, 1 out]
  }
  n82 = Build Array (concatenate)(w18, w43) -> (w42:refnum<vi>[])
  n83 = call "Adjust Dashboard Window.vi"("Sizing Refnums"=w32, "Size Constraints"=w36, "VI"=w45, "WIn Mode"=w17) -> ()  [unwired: 8 in]
  n84 = while {
    tunnel: [w185] -> _
    tunnel: w19 -> [w179]
    tunnel: w18 -> [w178]
    tunnel: w17 -> [w174]
    i -> [w185]
    stop <- FALSE stop-if-true
    n85 = local read "Vision - Dissabled Control"() -> (w176:u16)
    n86 = call <vilib>:"WPI_DashboardUpdateNames.vi"("Controls on Tab"=w178) -> ()  [unwired: 11 in]
    n87 = call <vilib>:"WPI_DashboardRetrieveStatusInfo.vi"("Vision"=w176, "Binding Refnum"=w179, "Window Mode Notifier"=w174, "TCP Cnx"="TCP") -> ("Power and Errors"=w180:T27, "Robot Metrics"=w183:T28, "Status Info"=w184:T29, "Control Info"=w181:T30, "Robot Mode"=w177:T11, "Process?"=w182:bool)  [unwired: 2 in]
    "Mode" <- w177
    n88 = case shown="True" w182 {
      tunnel: w184 -> [_ w212]
      tunnel: w183 -> [_ w211]
      tunnel: w181 -> [_ w210]
      tunnel: w180 -> [_ w209]
      tunnel: w177 -> [_ _]
      frame False {
        n89 = Wait (ms)(milliseconds to wait=u32 20) -> ()  [unwired: 1 out]
      }
      frame True {
        # "swap motors to match\ncharts and include battery"
        n90 = Unbundle By Name(w210) -> ("Joystick Values"=w199:T31)  [unwired: 1 out]
        n91 = Unbundle By Name(w209) -> ("Camera Addr"=→"Camera IP":string)  [unwired: 1 out]
        n92 = Unbundle By Name(w211) -> ()  [unwired: 1 out]
        n93 = Unbundle By Name(w212) -> ("Battery V"=w200:dbl)  [unwired: 1 out]
        n94 = call-poly <vilib>:"NT Read Value.vi"("Name"="RobotDrive Motors") -> ("Numeric Array"=w188:dbl[])  [unwired: 9 in, 1 out]
        n95 = Index Array(array=w188, index #1=1, index #4=0) -> (element #1=w204:dbl, element #2=w205:dbl, element #3=w203:dbl, element #4=w208:dbl)  [unwired: 2 in]
        n96 = Index Array(array=w199) -> (element #1=w198:T32, element #2=w193:T32)  [unwired: 2 in]
        n97 = call "Prepare Joystick Data for Displays.vi"("Joystick Values"=w193) -> ("Buttons"=→"JS2 Buttons":T33, "Z Axis"=→"JS2 Z":dbl, "Cartesian Data"=→"JS2 Graph":cluster{"X axis":dbl, "X axis":dbl}[])  [unwired: 8 in]
        n98 = call "Prepare Joystick Data for Displays.vi"("Joystick Values"=w198) -> ("Buttons"=→"JS1 Buttons":T33, "Z Axis"=→"JS1 Z":dbl, "Cartesian Data"=→"JS1 Graph":cluster{"X axis":dbl, "X axis":dbl}[])  [unwired: 8 in]
        n99 = Bundle("Numeric"=w203, "Numeric"=w204) -> (→"MotorChart R" →"MotorSliders R":cluster{"Numeric":dbl, "Numeric":dbl})  [unwired: 1 in]
        n100 = Bundle("Numeric"=w205, "Numeric"=w208, "Battery V"=w200) -> (→"MotorChart L" →"MotorSliders L":T8)  [unwired: 1 in]
      }
    }
    n101 = call-poly <vilib>:"NT Read Value.vi"("Name"="Auton Mode") -> ("String"=→"Auton Mode":string)  [unwired: 9 in, 1 out]
  }
  n102 = register-events(refnum<vi> refnum, w8) -> (reference out=w50:refnum<event-registration>, error out=w49:errorcluster)  [unwired: 2 in]
  n103 = property class="VI"() -> ("Panel"=w53:refnum<vi>)  [unwired: 2 in, 2 out]
  n104 = while {
    tunnel: w42 -> [w225]
    tunnel: w19 -> [w223]
    tunnel: [w221] -> _
    tunnel: u32 1000 ("milliseconds to wait") -> [w220]
    tunnel: w8 -> [w213]
    i -> [w221]
    stop <- FALSE stop-if-true
    n105 = local read "Rec Mode"() -> (w216:enum32{"Stop", "Record", "Playback"})
    n106 = Wait on Notification(notifier=w223, timeout in ms (-1)=w220) -> (notification=w222:string, timed out?=w218:bool)  [unwired: 2 in, 2 out]
    n107 = Equal?(x=w216, y=u16 2 ("Rec Mode")) -> (x = y?=w217:bool)
    n108 = Compound Arithmetic op=OR(invert w218, w217) -> (w219:bool)
    n109 = case shown="True" w219 {
      tunnel: w225 -> [_ w229]
      tunnel: w222 -> [_ w228]
      tunnel: "Dashboard" -> [_ w227]
      tunnel: w213 -> [_ w226]
      frame False {
      }
      frame True {
        n110 = call <vilib>:"Bind Controls to SmartDashboard.vi"("RPC ref"=w226, "Client Name"=w227, "Bound Control Refs"=w229, "Server IP Address"=w228) -> ()  [unwired: 8 in]
      }
    }
  }
  n111 = vi-ref "Playback Controls.vi"() -> (w51:refnum<vi>)
  n112 = call "Initialize Camera and CheckList.vi"("ListBox in"=w31) -> ("Cluster"=w57:cluster{"value":i32, "value":i32, "index":i32}, "Array"=w58:cluster{string[]}[], "File Refnum"=w56:T34)  [unwired: 8 in]
  n113 = disable-structure shown="Disabled" {
    disable-tunnel: w63 -> [w231 _]
    disable-tunnel: w1 -> [w230 _]
    frame Disabled {
      # "Loop 2. Receive camera images from Robot, update Mbps, fps, and do any processing or display"
      n114 = while {
        tunnel: w230 -> [w240]
        tunnel: w231 -> [_]
        tunnel: [w241] -> _
        i -> [w241]
        stop <- FALSE stop-if-true
        # "Optionally read the DB image,\nlog, or retrieve images from a\nlogged match"
        n115 = local read "Rec Mode"() -> (w235:enum32{"Stop", "Record", "Playback"})
        n116 = local read "Camera IP"() -> (w233:string)
        n117 = call <vilib>:"WPI_CameraRead MJPG for Dashboard.vi"("Camera Settings"="Camera Settings", "Rec Mode"=w235, "Camera IP"=w233, "Camera Mode"="Vision - Dissabled Control", "Refnum in"=w240) -> ("Active"=w238:bool, "Refnum out"=w239:T1, "FPS"=w237:dbl, "Bandwidth (Mbps)"=w232:dbl)  [unwired: 3 in]
        "Mbps" <- w232
        n118 = case shown="True" w238 {
          tunnel: w239 -> [_ w250]
          tunnel: w232 -> [_ w249]
          tunnel: w237 -> [_ w247]
          frame False {
            w243 = u32 1985280 ("Color Box")
            # "Sleep for 500ms"
            n119 = Bundle("Color Box"=w243, "Color Box"=w243) -> (w245:cluster{"Color Box":u32, "Color Box":u32})  [unwired: 1 out]
            n120 = Build Array(w245) -> (w244:cluster{"Color Box":u32, "Color Box":u32}[])
            n121 = property on="Mbps LED" class="Bool (strict)"("Colors [4]"=w244) -> ()  [unwired: 2 in, 2 out]
            n122 = Wait Until Next ms Multiple(millisecond multiple=u32 500) -> ()  [unwired: 1 out]
          }
          frame True {
            # "Here is where you would annotate,\npossibly process, and display the image"
            # "Update Mbps LED"
            n123 = call "IMAQ Clear Overlay"("Image"=w250) -> ("error out"=w254:errorcluster, "Image Out"=→"Camera Image":T1)  [unwired: 2 in, 7 out]
            n124 = case shown="Default" w249 {
              tunnel: [u32 6618880 ("Color Box") u32 16776722 ("Color Box") u32 16716800 ("Color Box")] -> w251
              frame Default {
              }
              frame 4, 5 {
              }
              frame 6.. {
              }
            }
            n125 = Unbundle By Name(w254) -> ("status"=w255:bool)
            n126 = Bundle("Color Box"=w251, "Color Box"=w251) -> (w253:cluster{"Color Box":u32, "Color Box":u32})  [unwired: 1 out]
            n127 = property on="Image Message" class="Str"("Visible"=w255) -> ()  [unwired: 2 in, 2 out]
            n128 = Build Array(w253) -> (w252:cluster{"Color Box":u32, "Color Box":u32}[])
            n129 = property on="Mbps LED" class="Bool (strict)"("Colors [4]"=w252) -> ()  [unwired: 2 in, 2 out]
            "fps" <- w247
          }
        }
      }
    }
    frame Enabled {
    }
  }
  n130 = property class="Pnl"(reference=w53) -> ("Panes[]"=w54:refnum<vi>[])  [unwired: 1 in, 2 out]
  n131 = property on="Camera Settings" class="Clust (strict)"("Val(Sgnl)"=w57) -> ()  [unwired: 2 in, 2 out]
  n132 = Index Array(array=w54) -> (element=w52:refnum<vi>)  [unwired: 1 in]
  n133 = control-ref of="Test Tree"() -> (w55:refnum<vi>)
  n134 = while {
    tunnel: w58 -> [w270]
    shift-right: [w269] -> _
    shift-left: w56 -> [w268]
    tunnel: [w267] -> _
    tunnel: w55 -> [w266]
    tunnel: w51 -> [w265]
    tunnel: w50 -> [w264]
    tunnel: w49 -> [_]
    tunnel: w45 -> [w263]
    tunnel: w8 -> [w262]
    tunnel: w6 -> [w261]
    shift-right: [w260] -> _
    shift-left: _ -> [w259]
    i -> [w267]
    stop <- FALSE stop-if-true
    n135 = event shown="[0] Timeout" {
      selector: w264 -> [_ _ _ _ _ _ _ _ _ _ _ _ _ _ _ _ _ _ _ _ _ _ _ _]
      dyn-events: [_ _ _ _ _ _ _ _ _ _ _ _ _ _ _ _ _ _ w579 _ _ _ _ _] -> _
      timeout: u32 60 ("milliseconds to wait") -> [_ _ _ _ _ _ _ _ _ _ _ _ _ _ _ _ _ _ _ _ _ _ _ _]
      tunnel: w266 -> [w283 _ _ _ _ _ _ _ _ _ _ _ _ _ _ _ _ _ _ _ _ _ _ _]
      tunnel: "Test Tree" -> [_ _ _ _ _ _ _ _ _ _ _ _ _ w542 w551 w554 w559 w568 _ _ _ _ _ _]
      tunnel: w270 -> [_ w321 _ _ _ _ _ _ _ _ _ w504 w535 _ _ _ _ _ _ _ _ _ _ _]
      tunnel: [w280 w320 w424 w430 w440 w444 w450 w462 w470 w476 w489 w503 w528 w541 w549 w553 w558 w567 w581 w597 w599 w607 w618 w623] -> w269
      tunnel: w268 -> [w280 w320 w424 w430 w440 w444 w450 w462 w470 w476 w489 w502 w528 w541 w549 w553 w558 w567 w581 w597 w599 w607 w618 w623]
      tunnel: w265 -> [_ _ _ _ _ _ _ _ _ _ _ _ _ _ _ _ _ _ w582 _ w602 _ _ _]
      tunnel: w263 -> [_ _ _ _ _ _ _ _ _ _ _ _ _ _ _ _ _ _ w577 _ _ _ _ _]
      tunnel: w262 -> [_ _ _ _ _ _ _ _ _ _ _ _ _ _ _ _ _ _ w573 _ _ _ _ _]
      tunnel: w261 -> [w275 _ _ _ _ _ w448 _ _ _ _ _ _ _ _ _ _ _ _ _ _ _ _ _]
      tunnel: [w274 w319 w423 w429 w439 w445 w446 w456 w467 w475 w488 w501 w527 w540 w548 w552 w557 w566 w572 w595 w598 w603 w611 w624] -> w260
      tunnel: w259 -> [w274 w319 w423 w429 w439 w445 w446 _ _ w475 w488 w501 w527 w540 w548 w552 w557 w566 w572 w595 w598 w603 w611 w624]
      event Timeout {
        n136 = event-data() -> ()  [unwired: 1 in, 1 out]
        n137 = local read "Mode"() -> (w277:T11)
        n138 = call <vilib>:"NT Read String.vi"("Name"="/TestMode/TestName") -> ("String"=w286:string)  [unwired: 9 in, 1 out]
        n139 = case shown="\"Test\"" "Dashboard Tab" {
          tunnel: w283 -> [_ w297 _ _]
          tunnel: "/TestMode/Automatic/" ("Name Pattern") -> [_ w296 _ _]
          tunnel: T35 [{"Operation"=enum."Clear", "Color Box"=14013909}, {"Operation"=enum."Clear", "Color Box"=14013909}, {"Operation"=enum."Clear", "Color Box"=14013909}, {"Operation"=enum."Clear", "Color Box"=14013909}, {"Operation"=enum."Update", "Color Box"=14013909}, {"Operation"=enum."Update", "Color Box"=16777215}, {"Operation"=enum."Clear", "Color Box"=14013909}, {"Operation"=enum."Clear", "Color Box"=14013909}, {"Operation"=enum."Clear", "Color Box"=14013909}] -> [_ w289 _ w306]
          tunnel: w277 -> [_ w288 _ w305]
          tunnel: u32[] [15790320, 15790320, 15790320, 15790320, 16777215, 16777215, 15790320, 15790320, 15790320] -> [_ _ _ w311]
          tunnel: w275 -> [_ _ _ w299]
          frame "Vision", Default {
          }
          frame "Test" {
            w295 = -2 ("Active Item:Row Number")
            n140 = Index Array(array=w289, index=w288) -> (element=w290:T39)
            n141 = Unbundle(w290) -> ("Operation"=w291:enum16{"Update", "Clear"}, "Color Box"=w292:u32)
            n142 = call <vilib>:"NT Read and Format Entries as Tree.vi"("Operation"=w291, "Name Pattern"=w296, "Tree Refnum"=w297) -> ()  [unwired: 7 in, 2 out]
            n143 = property on="Test Tree" class="Tree (strict)"("Active Item Row Number"=w295, "ActiveColNum"=w295, "CellBG"=w292, "Active Item Row Number"=-1 ("Active Item:Row Number"), "CellBG"=u32 5789784 ("Color Box")) -> ()  [unwired: 2 in, 2 out]
          }
          frame "Variables" {
            n144 = control-ref of="Tree"() -> (w298:refnum<vi>)
            n145 = call <vilib>:"NT Read and Format Entries as Tree.vi"("Tree Refnum"=w298) -> ()  [unwired: 9 in, 2 out]
          }
          frame "Comms" {
            w307 = u32 5789784 ("Color Box")
            w308 = T40 {"Row"=-1, "Column"=-2} ("Active Cell:Active Cell")
            w310 = T40 {"Row"=-2, "Column"=-2} ("Active Cell:Active Cell")
            n146 = Index Array(array=w311, index=w305) -> (element=w309:u32)
            n147 = Index Array(array=w306, index=w305) -> (element=w304:T39)
            n148 = Unbundle(w304) -> ("Operation"=w303:enum16{"Update", "Clear"})  [unwired: 1 out]
            n149 = local read "Command Selection"() -> (w302:i32)
            n150 = property on="Command Selection" class="MCListbox (strict)"("ActiveCell"=w310, "CellBG"=w309, "ActiveCell"=w308, "CellBG"=w307) -> ()  [unwired: 2 in, 2 out]
            n151 = call <vilib>:"WPI_DashboardUpdate RPC Info.vi"("Operation"=w303) -> ("update"=w301:bool, "commands"=w300:string[][])  [unwired: 9 in]
            n152 = property on="Command Selection" class="MCListbox (strict)"("ItemNames"=w300) -> ()  [unwired: 2 in, 2 out]
            n153 = property on="Command Params" class="Tbl (strict)"("Active Cell"=w310, "Cell BG Color"=w309, "Active Cell"=w308, "Cell BG Color"=w307) -> ()  [unwired: 2 in, 2 out]
            n154 = call <vilib>:"WPI_DashboardUpdate Command Params.vi"("Update"=w301, "NewVal"=w302, "Commands"=w300, "Param Tbl"=w299) -> ()  [unwired: 7 in, 1 out]
          }
        }
        n155 = case shown="\"\"" w286 {
          tunnel: "/TestMode/TestProgress" ("Name") -> [w313 _]
          tunnel: "/TestMode/TestProgressText" ("Name") -> [w312 _]
          frame Default {
            n156 = call <vilib>:"NT Read Number.vi"("Name"=w313) -> ("Numeric"=w314:dbl)  [unwired: 9 in, 1 out]
            n157 = call <vilib>:"NT Read String.vi"("Name"=w312) -> ("String"=w315:string)  [unwired: 9 in, 1 out]
            n158 = Bundle("Numeric"=w314, "String"=w315) -> (→"Progress":cluster{"Numeric":dbl, "String":string})  [unwired: 1 in]
          }
          frame "" {
            n159 = property on="Progress" class="Clust (strict)"("Visible"=FALSE) -> ()  [unwired: 2 in, 2 out]
            n160 = local write "Test Name"(u16 0) -> ()
          }
        }
        n161 = call <vilib>:"Connextion Info.vi"() -> ("Connected"=→"NT Connection":bool)  [unwired: 10 in, 1 out]
      }
      event "Test Tree": Value Change {
        # "Show appropriate\ncontrols"
        n162 = event-data() -> ("CtlRef"=w324:refnum<vi>, "NewVal"=w322:string)  [unwired: 1 in]
        n163 = call <vilib>:"WPI_UtilitiesGetTreeIOName.vi"("NewVal"=w322, "TreeControl in"=w324) -> ("I/O Name"=w325:string)  [unwired: 9 in]
        n164 = case shown="\"Analog Out\", \"Motor\", \"PWM\"" w325 {
          selector: w325 -> [_ w332 _ w354 w363 _]
          tunnel: w322 -> [_ _ w351 w353 _ w370]
          tunnel: w321 -> [_ _ _ _ _ w369]
          frame Default {
            w327 = FALSE ("Visible")
            w326 = FALSE ("Visible")
            n165 = property on="Motor" class="Clust (strict)"("Visible"=w326) -> ()  [unwired: 2 in, 2 out]
            n166 = property on="Test Ring" class="Ring (strict)"("Visible"=w326) -> ()  [unwired: 2 in, 2 out]
            n167 = property on="Rev/Fwd" class="Clust (strict)"("Visible"=w327) -> ()  [unwired: 2 in, 2 out]
            n168 = property on="On/Off" class="Bool (strict)"("Visible"=w327) -> ()  [unwired: 2 in, 2 out]
            n169 = property on="Test Slider" class="Slide (strict)"("Visible"=w327) -> ()  [unwired: 2 in, 2 out]
          }
          frame "Analog Out", "Motor", "PWM" {
            w333 = FALSE ("Visible")
            n170 = case shown="\"Analog Out\"" w332 {
              tunnel: [1.0 ("Value") -1.0 ("Value") 0.0 ("Value")] -> w331
              tunnel: [255.0 ("Value") 1.0 ("Value") 5.0 ("Value")] -> w330
              tunnel: [128.0 ("Value") 0.0 ("Value") 0.0 ("Value")] -> w329
              tunnel: [64.0 ("Value") 0.5 ("Value") 1.0 ("Value")] -> w328
              frame "PWM" {
              }
              frame "Motor", Default {
              }
              frame "Analog Out" {
              }
            }
            n171 = property on="Motor" class="Clust (strict)"("Visible"=TRUE) -> ()  [unwired: 2 in, 2 out]
            n172 = property on="Value" class="Slide (strict)"("Value"=w329, "Scale.Minimum"=w331, "Scale.Maximum"=w330, "Scale.Increment"=w328) -> ()  [unwired: 2 in, 2 out]
            n173 = property on="On/Off" class="Bool (strict)"("Visible"=w333) -> ()  [unwired: 2 in, 2 out]
            n174 = property on="Test Slider" class="Slide (strict)"("Visible"=w333) -> ()  [unwired: 2 in, 2 out]
            n175 = property on="Test Ring" class="Ring (strict)"("Visible"=w333) -> ()  [unwired: 2 in, 2 out]
            n176 = property on="Rev/Fwd" class="Clust (strict)"("Visible"=w333) -> ()  [unwired: 2 in, 2 out]
          }
          frame "Servo" {
            w349 = FALSE ("Visible")
            n177 = call <vilib>:"NT Read Number.vi"("Name"=w351) -> ("Numeric"=w350:dbl)  [unwired: 9 in, 1 out]
            n178 = property on="Test Slider" class="Slide (strict)"("Visible"=TRUE, "Scale.Maximum"=170.0 ("Scale.Range:Maximum")) -> ()  [unwired: 2 in, 2 out]
            n179 = local write "Test Slider"(w350) -> ()
            n180 = property on="Motor" class="Clust (strict)"("Visible"=w349) -> ()  [unwired: 2 in, 2 out]
            n181 = property on="Rev/Fwd" class="Clust (strict)"("Visible"=w349) -> ()  [unwired: 2 in, 2 out]
            n182 = property on="On/Off" class="Bool (strict)"("Visible"=w349) -> ()  [unwired: 2 in, 2 out]
            n183 = property on="Test Ring" class="Ring (strict)"("Visible"=w349) -> ()  [unwired: 2 in, 2 out]
          }
          frame "Relay", "Solenoid" {
            w352 = FALSE ("Visible")
            n184 = property on="Motor" class="Clust (strict)"("Visible"=w352) -> ()  [unwired: 2 in, 2 out]
            n185 = property on="Test Slider" class="Slide (strict)"("Visible"=w352) -> ()  [unwired: 2 in, 2 out]
            n186 = Search and Replace String(input string=w353, search string="/Value  **", replace string="/Direction") -> (result string=w359:string)  [unwired: 5 in, 3 out]
            n187 = property on="Test Ring" class="Ring (strict)"("Visible"=w352) -> ()  [unwired: 2 in, 2 out]
            n188 = call <vilib>:"NT Read String.vi"("Name"=w359) -> ("String"=w357:string)  [unwired: 9 in, 1 out]
            n189 = Equal?(x="Both directions", y=w357) -> (x = y?=w355:bool)
            n190 = Not(x=w355) -> (.not. x?=w356:bool)
            n191 = property on="Rev/Fwd" class="Clust (strict)"("Visible"=w355) -> ()  [unwired: 2 in, 2 out]
            n192 = property on="On/Off" class="Bool (strict)"("Visible"=w356, "Caption.Text"=w354) -> ()  [unwired: 2 in, 2 out]
          }
          frame "Compressor", "Digital Out" {
            w362 = FALSE ("Visible")
            # "Get direction and finish"
            n193 = property on="Motor" class="Clust (strict)"("Visible"=w362) -> ()  [unwired: 2 in, 2 out]
            n194 = property on="Test Slider" class="Slide (strict)"("Visible"=w362) -> ()  [unwired: 2 in, 2 out]
            n195 = property on="Test Ring" class="Ring (strict)"("Visible"=w362) -> ()  [unwired: 2 in, 2 out]
            n196 = property on="On/Off" class="Bool (strict)"("Visible"=TRUE, "Caption.Text"=w363) -> ()  [unwired: 2 in, 2 out]
            n197 = property on="Rev/Fwd" class="Clust (strict)"("Visible"=FALSE) -> ()  [unwired: 2 in, 2 out]
          }
          frame "Camera" {
            n198 = call <vilib>:"Get Last Path Segment.vi"("String in"=w370) -> ("String out"=w371:string)  [unwired: 10 in]
            n199 = property on="On/Off" class="Bool (strict)"("Visible"=FALSE) -> ()  [unwired: 2 in, 2 out]
            n200 = property on="Motor" class="Clust (strict)"("Visible"=FALSE) -> ()  [unwired: 2 in, 2 out]
            n201 = property on="Rev/Fwd" class="Clust (strict)"("Visible"=FALSE) -> ()  [unwired: 2 in, 2 out]
            n202 = case shown="\"White Balance  **\"" w371 {
              tunnel: w370 -> [w377 w386 w395 w404 w413 _ w419]
              tunnel: w369 -> [w375 w383 w392 w401 w410 _ _]
              frame "Size  **" {
                n203 = Index Array(array=w375) -> (element=w374:cluster{string[]})  [unwired: 1 in]
                n204 = call <vilib>:"NT Read String.vi"("Name"=w377) -> ("String"=w376:string)  [unwired: 9 in, 1 out]
                n205 = Unbundle(w374) -> (w372:string[])
                n206 = Match First String(2:w372, 3:w376) -> (0:w373:i32)  [unwired: 1 out]
                n207 = property on="Test Ring" class="Ring (strict)"("Value"=w373, "Strings []"=w372) -> ()  [unwired: 2 in, 2 out]
                n208 = property on="Test Ring" class="Ring (strict)"("Visible"=TRUE) -> ()  [unwired: 2 in, 2 out]
                n209 = property on="Test Slider" class="Slide (strict)"("Visible"=FALSE) -> ()  [unwired: 2 in, 2 out]
              }
              frame "White Balance  **" {
                n210 = Index Array(array=w383, index=1) -> (element=w384:cluster{string[]})
                n211 = call <vilib>:"NT Read String.vi"("Name"=w386) -> ("String"=w385:string)  [unwired: 9 in, 1 out]
                n212 = Unbundle(w384) -> (w381:string[])
                n213 = Match First String(2:w381, 3:w385) -> (0:w380:i32)  [unwired: 1 out]
                n214 = property on="Test Ring" class="Ring (strict)"("Value"=w380, "Strings []"=w381) -> ()  [unwired: 2 in, 2 out]
                n215 = property on="Test Ring" class="Ring (strict)"("Visible"=TRUE) -> ()  [unwired: 2 in, 2 out]
                n216 = property on="Test Slider" class="Slide (strict)"("Visible"=FALSE) -> ()  [unwired: 2 in, 2 out]
              }
              frame "Exposure  **" {
                n217 = Index Array(array=w392, index=2) -> (element=w393:cluster{string[]})
                n218 = call <vilib>:"NT Read String.vi"("Name"=w395) -> ("String"=w394:string)  [unwired: 9 in, 1 out]
                n219 = Unbundle(w393) -> (w389:string[])
                n220 = Match First String(2:w389, 3:w394) -> (0:w390:i32)  [unwired: 1 out]
                n221 = property on="Test Ring" class="Ring (strict)"("Value"=w390, "Strings []"=w389) -> ()  [unwired: 2 in, 2 out]
                n222 = property on="Test Ring" class="Ring (strict)"("Visible"=TRUE) -> ()  [unwired: 2 in, 2 out]
                n223 = property on="Test Slider" class="Slide (strict)"("Visible"=FALSE) -> ()  [unwired: 2 in, 2 out]
              }
              frame "Exposure Priority  **" {
                n224 = Index Array(array=w401, index=3) -> (element=w402:cluster{string[]})
                n225 = call <vilib>:"NT Read String.vi"("Name"=w404) -> ("String"=w403:string)  [unwired: 9 in, 1 out]
                n226 = Unbundle(w402) -> (w398:string[])
                n227 = Match First String(2:w398, 3:w403) -> (0:w399:i32)  [unwired: 1 out]
                n228 = property on="Test Ring" class="Ring (strict)"("Value"=w399, "Strings []"=w398) -> ()  [unwired: 2 in, 2 out]
                n229 = property on="Test Ring" class="Ring (strict)"("Visible"=TRUE) -> ()  [unwired: 2 in, 2 out]
                n230 = property on="Test Slider" class="Slide (strict)"("Visible"=FALSE) -> ()  [unwired: 2 in, 2 out]
              }
              frame "Color Enable  **" {
                n231 = Index Array(array=w410, index=4) -> (element=w411:cluster{string[]})
                n232 = call <vilib>:"NT Read String.vi"("Name"=w413) -> ("String"=w412:string)  [unwired: 9 in, 1 out]
                n233 = Unbundle(w411) -> (w407:string[])
                n234 = Match First String(2:w407, 3:w412) -> (0:w408:i32)  [unwired: 1 out]
                n235 = property on="Test Ring" class="Ring (strict)"("Value"=w408, "Strings []"=w407) -> ()  [unwired: 2 in, 2 out]
                n236 = property on="Test Ring" class="Ring (strict)"("Visible"=TRUE) -> ()  [unwired: 2 in, 2 out]
                n237 = property on="Test Slider" class="Slide (strict)"("Visible"=FALSE) -> ()  [unwired: 2 in, 2 out]
              }
              frame Default {
                n238 = property on="Test Ring" class="Ring (strict)"("Visible"=FALSE) -> ()  [unwired: 2 in, 2 out]
                n239 = property on="Test Slider" class="Slide (strict)"("Visible"=FALSE) -> ()  [unwired: 2 in, 2 out]
              }
              frame "Brightness  **", "Color Level  **", "Compression  **", "FPS  **", "Sharpness  **" {
                n240 = call <vilib>:"NT Read Number.vi"("Name"=w419) -> ("Numeric"=w418:dbl)  [unwired: 9 in, 1 out]
                n241 = local write "Test Slider"(w418) -> ()
                n242 = property on="Test Slider" class="Slide (strict)"("Visible"=TRUE, "Scale.Maximum"=100.0 ("Scale.Range:Maximum")) -> ()  [unwired: 2 in, 2 out]
                n243 = property on="Test Ring" class="Ring (strict)"("Visible"=FALSE) -> ()  [unwired: 2 in, 2 out]
              }
            }
          }
        }
        n244 = property on="Progress" class="Clust (strict)"("Visible"=FALSE) -> ()  [unwired: 2 in, 2 out]
      }
      event "Test Name": Mouse Enter {
        # "Populate the ring with the list of tests"
        n245 = event-data() -> ()  [unwired: 1 in, 1 out]
        n246 = call <vilib>:"NT Read String Array.vi"("Name"="/TestMode/TestList") -> ("String Array"=w428:string[])  [unwired: 9 in, 1 out]
        n247 = Build Array (concatenate)("Select the test to run...", w428) -> (w427:string[])
        n248 = property on="Test Name" class="Ring (strict)"("Strings []"=w427) -> ()  [unwired: 2 in, 2 out]
      }
      event "Test Name": Value Change {
        w431 = FALSE ("Visible")
        # "Tell the robot the test name to run"
        n249 = event-data() -> ("NewVal"=w435:u16)  [unwired: 1 in]
        n250 = property on="Test Name" class="Ring (strict)"() -> ("Strings []"=w436:string[])  [unwired: 2 in, 2 out]
        n251 = local write "Progress"(T15 {"Test Progress"=0, "Test Progress Text"=""} ("Progress")) -> ()
        n252 = Index Array(array=w436, index=w435) -> (element=w434:string)
        n253 = call <vilib>:"NT Write String.vi"("String"=w434, "Name"="/TestMode/TestName") -> ()  [unwired: 9 in, 1 out]
        n254 = property on="Progress" class="Clust (strict)"("Visible"=TRUE) -> ()  [unwired: 2 in, 2 out]
        n255 = property on="Motor" class="Clust (strict)"("Visible"=w431) -> ()  [unwired: 2 in, 2 out]
        n256 = property on="Test Slider" class="Slide (strict)"("Visible"=w431) -> ()  [unwired: 2 in, 2 out]
        n257 = property on="On/Off" class="Bool (strict)"("Visible"=w431) -> ()  [unwired: 2 in, 2 out]
        n258 = property on="Rev/Fwd" class="Clust (strict)"("Visible"=w431) -> ()  [unwired: 2 in, 2 out]
        n259 = property on="Test Ring" class="Ring (strict)"("Visible"=w431) -> ()  [unwired: 2 in, 2 out]
      }
      event "Select Auto": Mouse Enter {
        # "Populate the combo box with the list of autonomous options"
        n260 = event-data() -> ()  [unwired: 1 in, 1 out]
        n261 = call <vilib>:"NT Read String Array.vi"("Name"="Auto List") -> ("String Array"=w438:string[])  [unwired: 9 in, 1 out]
        n262 = property on="Select Auto" class="CmbBox"("Strings[]"=w438) -> ()  [unwired: 2 in, 2 out]
      }
      event "Select Auto": Value Change {
        # "User modified the Auto Selection. Write to NT variable so robot knows."
        n263 = event-data() -> ("NewVal"=w442:string)  [unwired: 1 in]
        n264 = call <vilib>:"NT Write String.vi"("String"=w442, "Name"="Auto Selector") -> ()  [unwired: 9 in, 1 out]
      }
      event "Command Selection": Value Change {
        # "Get the params and show in table"
        n265 = event-data() -> ("NewVal"=w449:i32)  [unwired: 1 in]
        n266 = property on="Command Selection" class="MCListbox (strict)"() -> ("ItemNames"=w447:string[][])  [unwired: 2 in, 2 out]
        n267 = call <vilib>:"WPI_DashboardUpdate Command Params.vi"("NewVal"=w449, "Commands"=w447, "Param Tbl"=w448) -> ()  [unwired: 8 in, 1 out]
      }
      event "Execute Command": Value Change {
        # "Started one, Unique ID holds\nresponse"
        n268 = event-data() -> ()  [unwired: 1 in, 1 out]
        n269 = property on="Command Selection" class="MCListbox (strict)"() -> ("ItemNames"=w461:string[][])  [unwired: 2 in, 2 out]
        n270 = Index Array(array=w461, index (row)="Command Selection", index (col)=0) -> (element=w459:string)
        n271 = call <vilib>:"Invoke Commands.vi"("Command Params"="Command Params", "Function Name"=w459) -> ("Params"=w455:u8, "Started"=w454:bool)  [unwired: 7 in, 1 out]
        n272 = Array Subset(array="Command Params", length (row)=w455) -> (w456:string[][])  [unwired: 3 in]
        n273 = Select(t="Executing" ("Cmd Status"), s=w454, f="" ("Cmd Status")) -> (s? t:f=→"Cmd Status":string)
      }
      event "Command Selection": Double Click {
        n274 = event-data() -> ("Row"=w471:i32)  [unwired: 1 in]
        n275 = property on="Command Selection" class="MCListbox (strict)"() -> ("ItemNames"=w474:string[][])  [unwired: 2 in, 2 out]
        n276 = local read "Command Params"() -> (w469:string[][])
        n277 = Index Array(array=w474, index (row)=w471, index (col)=0) -> (element=w472:string)
        n278 = call <vilib>:"Invoke Commands.vi"("Command Params"=w469, "Function Name"=w472) -> ("Params"=w468:u8, "Started"=w463:bool)  [unwired: 7 in, 1 out]
        n279 = Array Subset(array=w469, length (row)=w468) -> (w467:string[][])  [unwired: 3 in]
        n280 = Select(t="Executing" ("Cmd Status"), s=w463, f="" ("Cmd Status")) -> (s? t:f=w464:string)
        n281 = local write "Cmd Status"(w464) -> ()
      }
      event "CheckList": Double Click {
        # "Shift clears all"
        # "Update symbols on the listbox"
        n282 = event-data() -> ("PlatMods.Shift"=w477:bool, "Row"=w479:i32)  [unwired: 1 in]
        n283 = case shown="True" w477 {
          tunnel: w479 -> [w483 _]
          tunnel: 1 -> [w482 _]
          frame False {
            n284 = property on="CheckList" class="LstBox (strict)"() -> ("Item Symbols"=w481:i32[])  [unwired: 2 in, 2 out]
            n285 = Replace Array Subset(array=w481, new element=w482, index=w483) -> (w480:i32[])
            n286 = property on="CheckList" class="LstBox (strict)"("Item Symbols"=w480) -> ()  [unwired: 2 in, 2 out]
          }
          frame True {
            w484 = 0 ("Top Row")
            n287 = property on="CheckList" class="LstBox (strict)"() -> ("Number of Rows"=w486:u32)  [unwired: 2 in, 2 out]
            n288 = Initialize Array(0, w486) -> (w485:i32[])
            n289 = property on="CheckList" class="LstBox (strict)"("Top Row"=w484, "Value"=w484, "Item Symbols"=w485) -> ()  [unwired: 2 in, 2 out]
          }
        }
      }
      event "CheckList": Key Down {
        # "Update symbols on the listbox\nLeft and right keys check and uncheck"
        n290 = event-data() -> ("VKey"=w491:T36)  [unwired: 1 in]
        n291 = case shown="\"Left\", \"Right\"" w491 {
          selector: w491 -> [w496 _]
          tunnel: eventvkey."Left" ("VKey") -> [w494 _]
          frame "Left", "Right" {
            n292 = Equal?(x=w494, y=w496) -> (x = y?=w495:bool)
            n293 = Select(t=0, s=w495, f=1) -> (s? t:f=w497:i32)
            n294 = property on="CheckList" class="LstBox (strict)"() -> ("Item Symbols"=w500:i32[])  [unwired: 2 in, 2 out]
            n295 = Replace Array Subset(array=w500, new element=w497, index="CheckList") -> (w499:i32[])
            n296 = property on="CheckList" class="LstBox (strict)"("Item Symbols"=w499) -> ()  [unwired: 2 in, 2 out]
          }
          frame Default {
          }
        }
      }
      event "DB Camera Config": Value Change {
        # "Show or hide the cluster of controls, store in ini file"
        n297 = event-data() -> ("NewVal"=w505:bool)  [unwired: 1 in]
        n298 = case shown="False" w505 {
          tunnel: w504 -> [w514 _]
          tunnel: [w507 w525] -> w503
          tunnel: w502 -> [w506 w525]
          frame False {
            w521 = "Camera"
            w524 = FALSE ("Visible")
            n299 = local read "Camera Settings"() -> (w513:T7)
            n300 = Index Array(array=w514) -> (element=w517:cluster{string[]})  [unwired: 1 in]
            n301 = Unbundle(w513) -> ("Frame Rate"=w512:i32, "Compression"=w511:i32, "Size"=w515:u16)
            n302 = Unbundle(w517) -> (w516:string[])
            n303 = Index Array(array=w516, index=w515) -> (element=w510:string)
            n304 = call-poly <vilib>:"Write Key.vi"("section"=w521, "value"=w510, "key"="Size", "refnum"=w506) -> ("refnum out"=w523:T34)  [unwired: 2 in, 5 out]
            n305 = call-poly <vilib>:"Write Key.vi"("section"=w521, "value"=w512, "key"="FrameRate", "refnum"=w523) -> ("refnum out"=w522:T34)  [unwired: 1 in, 6 out]
            n306 = property on="Camera Settings" class="Clust (strict)"("Visible"=w524) -> ()  [unwired: 2 in, 2 out]
            n307 = local write "DB Camera Config"(w524) -> ()
            n308 = call-poly <vilib>:"Write Key.vi"("section"=w521, "value"=w511, "key"="Compression", "refnum"=w522) -> ("refnum out"=w508:T34)  [unwired: 1 in, 6 out]
            n309 = call <vilib>:"Close Config Data.vi"("refnum"=w508) -> ("file path"=w509:path)  [unwired: 2 in, 8 out]
            n310 = call <vilib>:"Open Config Data.vi"("configuration file path"=w509) -> ("refnum"=w507:T34)  [unwired: 8 in, 2 out]
          }
          frame True {
            n311 = property on="Camera Settings" class="Clust (strict)"("Visible"=TRUE) -> ()  [unwired: 2 in, 2 out]
          }
        }
      }
      event "Camera Settings": Value Change {
        # "Update summary string when any elements of DB camera change"
        n312 = event-data() -> ("NewVal"=w539:T7)  [unwired: 1 in]
        n313 = Index Array(array=w535) -> (element=w534:cluster{string[]})  [unwired: 1 in]
        n314 = Unbundle(w539) -> ("Frame Rate"=w530:i32, "Compression"=w529:i32, "Size"=w532:u16)
        n315 = Unbundle(w534) -> (w533:string[])
        n316 = Index Array(array=w533, index=w532) -> (element=w531:string)
        n317 = Format Into String(format string="%s   %dfps   %d%%", w531, w530, w529) -> (resulting string=w536:string)  [unwired: 2 in, 1 out]
        n318 = Build Array(w536) -> (w537:string[])
        n319 = property on="DB Camera Config" class="Bool (strict)"("Strings [4]"=w537) -> ()  [unwired: 2 in, 2 out]
      }
      event "Motor.Enable": Value Change {
        # "When the test mode otor enable helper is set, update that\ntree row item's value"
        n320 = event-data() -> ("NewVal"=w546:bool)  [unwired: 1 in]
        n321 = Unbundle("Motor") -> ("Value"=w545:dbl)  [unwired: 1 out]
        n322 = Select(t=w545, s=w546, f=0.0) -> (s? t:f=w543:dbl)
        n323 = call <vilib>:"NT Write Number.vi"("Numeric"=w543, "Name"=w542) -> ()  [unwired: 9 in, 1 out]
      }
      event "Test Slider": Value Change {
        # "When the test mode slider helper is set, update that\ntree row item's value"
        n324 = event-data() -> ("NewVal"=w550:dbl)  [unwired: 1 in]
        n325 = call <vilib>:"NT Write Number.vi"("Numeric"=w550, "Name"=w551) -> ()  [unwired: 9 in, 1 out]
      }
      event "On/Off": Value Change {
        # "When the test mode on/off helper value is set, update that\ntree row item's value"
        n326 = event-data() -> ("NewVal"=w556:bool)  [unwired: 1 in]
        n327 = Boolean To (0,1)(Boolean=w556) -> (0, 1=w555:i16)
        n328 = call <vilib>:"NT Write Number.vi"("Numeric"=w555, "Name"=w554) -> ()  [unwired: 9 in, 1 out]
      }
      event "Rev/Fwd": Value Change {
        # "When the test mode helper value for relays is set, update that\ntree row item's value"
        n329 = event-data() -> ("NewVal.Forward"=w565:bool, "NewVal.Reverse"=w564:bool)  [unwired: 1 in]
        n330 = Boolean To (0,1)(Boolean=w565) -> (0, 1=w561:i16)
        n331 = Boolean To (0,1)(Boolean=w564) -> (0, 1=w563:i16)
        n332 = Negate(x=w563) -> (-x=w562:i16)
        n333 = Add(x=w561, y=w562) -> (x+y=w560:i16)
        n334 = call <vilib>:"NT Write Number.vi"("Numeric"=w560, "Name"=w559) -> ()  [unwired: 9 in, 1 out]
      }
      event "Test Ring": Value Change {
        # "When a test mode helper value is selected from the ring,\nset the tree item's variable to the string value"
        n335 = event-data() -> ("NewVal"=w570:u16)  [unwired: 1 in]
        n336 = property on="Test Ring" class="Ring (strict)"() -> ("Strings []"=w571:string[])  [unwired: 2 in, 2 out]
        n337 = Index Array(array=w571, index=w570) -> (element=w569:string)
        n338 = call <vilib>:"NT Write String.vi"("String"=w569, "Name"=w568) -> ()  [unwired: 9 in, 1 out]
      }
      event "Rec Mode": Value Change {
        # "Update globals for recording mode and path to read log from.\nClear when logging and let NetworkTables set path for vision to\nuse."
        n339 = event-data() -> ("NewVal"=w583:enum32{"Stop", "Record", "Playback"})  [unwired: 1 in]
        n340 = global write "WPI_DashboardLogging Global.vi" "Logging Filename"(path "") -> ()
        n341 = global write "WPI_DashboardLogging Global.vi" "Recording"(w583) -> ()
        n342 = case shown="\"Playback\"" w583 {
          tunnel: w582 -> [_ w585 w594]
          tunnel: [_ _ w593] -> w579
          tunnel: [_ _ w592] -> _
          tunnel: w577 -> [_ _ w590]
          tunnel: cluster{i32, i32} {-250, 170} -> [_ _ w589]
          tunnel: [_ _ T37 {"Image Size"=TRUE, "Image Type"=TRUE, "Pixel Value"=TRUE, "ROI Information"=TRUE, "Zoom Factor"=FALSE} ("Image Information Shown:All Elements")] -> w575
          tunnel: [_ _ TRUE ("Zoom Factor")] -> w574
          tunnel: w573 -> [_ _ w586]
          frame Default {
          }
          frame "Stop", "Record" {
            # "Place Window too"
            n343 = invoke class="VI" method="FP.Close"(reference=w585) -> (reference out=w584:refnum<vi>)  [unwired: 2 in, 2 out]
            n344 = invoke class="VI" method="Abort VI"(reference=w584) -> ()  [unwired: 2 in, 3 out]
          }
          frame "Playback" {
            n345 = call "Open Playback Panel.vi"("Offset"=w589, "DB VI Ref"=w590, "Playback in"=w594) -> ("Playback out"=w591:refnum<vi>)  [unwired: 8 in]
            n346 = register-events(w591, w586) -> (reference out=w593:refnum<event-registration>, error out=w592:errorcluster)  [unwired: 2 in]
          }
        }
        n347 = property on="Camera Image" class="ImageControl"("Image Information Shown"=w575, "Image Information Visible"=w574) -> ()  [unwired: 2 in, 2 out]
        n348 = call <vilib>:"WPI_DashboardNT Log FieldName Cache.vi"("Operation"=enum16{"Lookup/Add", "Index", "Clear"}."Clear") -> ()  [unwired: 8 in, 3 out]
      }
      event Panel Close {
        w596 = enum32{"Stop", "Record", "Playback"}."Stop" ("Rec Mode")
        # "Playback window has been closed, abort"
        n349 = event-data() -> ()  [unwired: 1 in, 4 out]
        n350 = local write "Rec Mode"(w596) -> ()
        n351 = global write "WPI_DashboardLogging Global.vi" "Recording"(w596) -> ()
      }
      event Panel Close {
        # "Abort playback window and ourself"
        n352 = event-data() -> ()  [unwired: 1 in, 4 out]
        n353 = invoke class="VI" method="FP.Close"(reference=w602) -> (reference out=w601:refnum<vi>)  [unwired: 2 in, 2 out]
        n354 = invoke class="VI" method="Abort VI"(reference=w601) -> (error out=w600:errorcluster)  [unwired: 2 in, 2 out]
        n355 = invoke class="VI" method="Abort VI"(error in=w600) -> ()  [unwired: 2 in, 3 out]
      }
      event User Event {
        n356 = event-data() -> ("IDs"=w610:cluster{"RPC field ID":u16, "Unique ID":u16}, "String"=w609:string)  [unwired: 1 in]
        n357 = Bundle("IDs"=w610, "String"=w609) -> (w608:T18)  [unwired: 1 in]
        n358 = call <vilib>:"Retrieve RPC Response.vi"("RPC Response"=w608) -> ("Output"=w605:string[][])  [unwired: 10 in]
        n359 = Build Array (concatenate)(w603, w605) -> (w604:string[][])
        n360 = local write "Command Params"(w604) -> ()
        n361 = local write "Cmd Status"("" ("Cmd Status")) -> ()
      }
      event "Vision - Dissabled Control": Value Change {
        # "Enable/Disable Compression slider.\nHW USB is hard-coded into the camera"
        n362 = event-data() -> ("NewVal"=w617:u16)  [unwired: 1 in]
        n363 = Equal?(x=w617, y=u32 2 ("milliseconds to wait")) -> (x = y?=w615:bool)
        n364 = Select(t=T38."Disabled and Grayed Out" ("Disabled"), s=w615, f=T38."Enabled" ("Disabled")) -> (s? t:f=w612:T38)
        n365 = property on="Compression" class="Slide (strict)"("DisabledEnum"=w612) -> ()  [unwired: 2 in, 2 out]
      }
      event "Tree": Double Click {
        n366 = event-data() -> ("PlatMods"=w622:T41, "Tag"=w621:string)  [unwired: 1 in]
        n367 = Unbundle(w622) -> ("Shift"=w620:bool)  [unwired: 4 out]
        n368 = Not(x=w620) -> (.not. x?=w619:bool)
        n369 = call <vilib>:"NT Update Persistence.vi"("Persistence"=w619, "Name"=w621) -> ()  [unwired: 9 in, 1 out]
      }
    }
  }
  n370 = while {
    tunnel: w52 -> [w626]
    i -> [w629]
    stop <- FALSE stop-if-true
    n371 = Wait (ms)(milliseconds to wait=u32 100) -> ()  [unwired: 1 out]
    n372 = case shown="\"Playback\"" "Rec Mode" {
      tunnel: w629 -> [_ _ w644]
      tunnel: [u32 2829099 ("Base Color") u32 11141120 ("Target Color") w633] -> w625
      frame "Stop", Default {
        # "Reset the color, extra updates don't cost much"
      }
      frame "Record" {
      }
      frame "Playback" {
        # "Playback"
        n373 = Quotient & Remainder(x=w644, y=u32 50 ("milliseconds to wait")) -> (x-y*floor(x/y)=w640:u32)  [unwired: 1 out]
        n374 = Divide(x=w640, y=u32 50 ("milliseconds to wait")) -> (x/y=w637:dbl)
        n375 = Multiply(x=6.283185307179586, y=w637) -> (x*y=w642:dbl)
        n376 = Sine(x=w642) -> (sin(x)=w641:dbl)
        n377 = Absolute Value(x=w641) -> (abs(x)=w634:dbl)
        n378 = call "Interpolate RGB Color.vi"("Proportion"=w634, "Target Color"=u32 30976, "Base Color"=u32 2829099) -> ("Result Color"=w633:u32)  [unwired: 8 in]
      }
    }
    n379 = property class="Pane"(reference=w626, "PaneColor"=w625) -> ()  [unwired: 1 in, 2 out]
  }
  n380 = local write "Dashboard Tab"(T4."Vision" ("Dashboard Tab")) -> ()
  n381 = property on="On/Off" class="Bool (strict)"("Visible"=w20) -> ()  [unwired: 2 in, 2 out]
  n382 = property on="Motor" class="Clust (strict)"("Visible"=w20) -> ()  [unwired: 2 in, 2 out]
  n383 = property on="Progress" class="Clust (strict)"("Visible"=w20) -> ()  [unwired: 2 in, 2 out]
  n384 = property on="Test Ring" class="Ring (strict)"("Visible"=w20) -> ()  [unwired: 2 in, 2 out]
  n385 = property on="Rev/Fwd" class="Clust (strict)"("Visible"=w20) -> ()  [unwired: 2 in, 2 out]
  n386 = property on="Camera Settings" class="Clust (strict)"("Visible"=w20) -> ()  [unwired: 2 in, 2 out]
  n387 = while {
    tunnel: u16 1741 ("timeout ms (25000)") -> [w646]
    stop <- FALSE stop-if-true
    n388 = TCP Create Listener(10:w646) -> (0:w645:errorcluster, 3:w647:refnum<k5>)  [unwired: 4 in, 1 out]
    n389 = case shown="No Error" w645 {
      selector: w645 -> [w649 _]
      tunnel: w647 -> [w650 _]
      frame No Error {
        n390 = while {
          tunnel: w650 -> [w653]
          tunnel: w649 -> [w652]
          stop <- FALSE stop-if-true
          n391 = TCP Wait On Listener(8:w652, 11:w653) -> (0:w654:errorcluster, 4:w655:refnum<k5>)  [unwired: 2 in, 3 out]
          n392 = local write "TCP"(w655) -> ()
          n393 = case shown="No Error" w654 {
            frame No Error {
            }
            frame Error {
              n394 = Wait (ms)(milliseconds to wait=u32 1000) -> ()  [unwired: 1 out]
            }
          }
        }
      }
      frame Error {
        n395 = Wait (ms)(milliseconds to wait=u32 1000) -> ()  [unwired: 1 out]
      }
    }
  }
  n396 = local write "DB Camera Config"(w20) -> ()
  n397 = local write "Command Params"(string[][] [] ("Command Params")) -> ()
  n398 = global write "WPI_DashboardLogging Global.vi" "Recording"(w46) -> ()
  n399 = local write "Command Selection"(u16 0 ("milliseconds to wait")) -> ()
  n400 = local write "Rec Mode"(w46) -> ()
